vi "DL-SMART-MS-Modify-05-25-5.0.vi"() -> ()   [LabVIEW 2013]
uses:
  <vilib>/Utility/file.llb/Read From Spreadsheet File (DBL).vi
  <vilib>/Utility/file.llb/Write To Spreadsheet File (DBL).vi
  <vilib>/vision/driver/NI_Vision_Acquisition_Software.lvlib
  <resource>/objmgr/imaqdx.rc
panel:
  in  "Shots/Point":i32=100
  in  "chamber in":bool caption="TakeMS"
  in  "chamber out":bool caption="TakeMS"
  out "Mass Spectrum (质谱图)":cluster{i32[], dbl[]}(graph)
  out "Image":T1(plugin-control)
  in  "Laser parameter":T3
  in  "ADC parameter":T4
  in  "ShutDownSystem":bool
  out "TenAccumulate":cluster{"MassX":dbl[], "TenScans":sgl[]}
  in  "ADC reference":refnum<vi>
  in  "SetLaserEnergy":dbl(slide) min=0.0 max=50.0 scale=0.0..20.0
  in  "LaserHV":u8=50 min=1 max=100
  in  "频率/Hz":u8=60
  out "plat zeroed":bool
  out "ADC aquiring":bool
  out "motor moving":bool
  out "busy":bool
  out "Pul.HV-Real":dbl
  in  "ReportResult":bool
  out "Identify Spcetrum":cluster{"all rows":dbl[], "all rows":dbl[]}[](graph)=[{"all rows"=array[50131 elements], "all rows"=array[50131 elements]}, {"all rows"=array[360 elements], "all rows"=[0.0, -15.85746, 0.0, 0.0, -4.11823, 0.0, 0.0, -20.55303, 0.0, 0.0, -3.65583, 0.0, 0.0, -2.69345, 0.0, 0.0, -4.4706, 0.0, 0.0, -6.07537, 0.0, 0.0, -4.25015, 0.0, 0.0, -6.95758, 0.0, 0.0, -2.04252, 0.0, 0.0, -7.70754, 0.0, 0.0, -4.28864, 0.0, 0.0, -4.00869, 0.0, 0.0, -4.47517, 0.0, 0.0, -14.21368, 0.0, 0.0, -6.66072, 0.0, 0.0, -6.50078, 0.0, 0.0, -3.75903, 0.0, 0.0, -17.29715, 0.0, 0.0, -6.92254, 0.0, 0.0, -2.52353, 0.0, 0.0, -3.06405, 0.0, 0.0, -16.54211, 0.0, 0.0, -5.10076, 0.0, 0.0, -8.01669, 0.0, 0.0, -40.71695, 0.0, 0.0, -4.03763, 0.0, 0.0, -3.14159, 0.0, 0.0, -2.79298, 0.0, 0.0, -13.41979, 0.0, 0.0, -7.6464, 0.0, 0.0, -6.18956, 0.0, 0.0, -2.44901, 0.0, 0.0, -5.1704, 0.0, 0.0, -3.62455, 0.0, 0.0, -6.443, 0.0, 0.0, -24.18432, 0.0, 0.0, -37.78631, 0.0, 0.0, -4.28528, 0.0, 0.0, -3.21654, 0.0, 0.0, -3.13522, 0.0, 0.0, -4.8477, 0.0, 0.0, -3.80614, 0.0, 0.0, -8.10386, 0.0, 0.0, -2.86382, 0.0, 0.0, -17.8978, 0.0, 0.0, -4.74503, 0.0, 0.0, -9.4855, 0.0, 0.0, -5.75364, 0.0, 0.0, -80.29859, 0.0, 0.0, -5.18928, 0.0, 0.0, -28.13783, 0.0, 0.0, -6.84449, 0.0, 0.0, -4.07742, 0.0, 0.0, -2.99391, 0.0, 0.0, -4.60838, 0.0, 0.0, -3.257, 0.0, 0.0, -5.79015, 0.0, 0.0, -24.98325, 0.0, 0.0, -4.30828, 0.0, 0.0, -5.54625, 0.0, 0.0, -5.47663, 0.0, 0.0, -100.0001, 0.0, 0.0, -21.11295, 0.0, 0.0, -12.03347, 0.0, 0.0, -6.35092, 0.0, 0.0, -4.71483, 0.0, 0.0, -6.58836, 0.0, 0.0, -3.41548, 0.0, 0.0, -3.10072, 0.0, 0.0, -4.79955, 0.0, 0.0, -4.88109, 0.0, 0.0, -32.02295, 0.0, 0.0, -20.17071, 0.0, 0.0, -9.63953, 0.0, 0.0, -8.63946, 0.0, 0.0, -6.018, 0.0, 0.0, -6.3389, 0.0, 0.0, -14.67808, 0.0, 0.0, -6.22948, 0.0, 0.0, -4.9166, 0.0, 0.0, -44.64096, 0.0, 0.0, -5.6163, 0.0, 0.0, -8.56872, 0.0, 0.0, -11.1186, 0.0, 0.0, -4.42493, 0.0, 0.0, -15.45284, 0.0, 0.0, -2.99091, 0.0, 0.0, -18.05376, 0.0, 0.0, -3.06669, 0.0, 0.0, -35.88844, 0.0, 0.0, -19.12645, 0.0, 0.0, -3.20878, 0.0, 0.0, -2.61247, 0.0, 0.0, -7.79975, 0.0, 0.0, -5.8874, 0.0, 0.0, -5.7487, 0.0, 0.0, -5.43834, 0.0, 0.0, -21.69908, 0.0, 0.0, -64.96584, 0.0, 0.0, -5.77762, 0.0, 0.0, -5.55465, 0.0, 0.0, -4.62119, 0.0, 0.0, -3.61176, 0.0, 0.0, -6.99332, 0.0, 0.0, -4.34549, 0.0, 0.0, -15.09003, 0.0, 0.0, -6.25437, 0.0, 0.0, -21.85243, 0.0, 0.0, -13.24381, 0.0, 0.0, -3.94672, 0.0, 0.0, -3.90192, 0.0, 0.0, -11.14967, 0.0, 0.0, -83.69183, 0.0, 0.0, -11.19559, 0.0, 0.0, -7.83445, 0.0, 0.0, -3.14763, 0.0, 0.0, -6.44728, 0.0, 0.0, -5.69155, 0.0, 0.0, -4.00216, 0.0]}]
  in  "IdentifyMS":bool
  in  "Identification Record (鉴定记录表)":i32(listbox)=6
  in  "Identification Results (单靶鉴定结果)":i32(listbox)=2
  in  "HVEnable":bool
  out "执行进度栏":u8(slide) caption="Vaccum" scale=0.0..1.0
  out "GateClose":bool
  out "LaserOK":bool
  out "HV-OK":bool
  out "Vacuum-OK":bool
  in  "Tab Control":T5(tab)
  in  "helix-Zeta-Step":dbl=100.0
  in  "helix-b":dbl=0.2
  in  "AcquireMS-Methods":u8(ring) items=["SinglePoint", "Multipoints", "MultiTar"]
  in  "MCPHV-Set":dbl=1400.0 min=0.0 max=1600.0
  in  "LensHV-Set":dbl=8000.0 min=0.0 max=10000.0
  in  "Tar.HV-Set":dbl=18010.0 min=0.0 max=20000.0
  in  "Pul.HV-Set":dbl=1400.0 min=0.0 max=2000.0
  in  "PulseDelay":dbl
  in  "ADCFreq":dbl
  in  "CH1_Coupling":u64(ring)=2 items=["Volt DC"=1, "Volt AC"=2, "Ampere DC"=4, "Ampere AC"=8, "Ohm"=16]
  in  "Channel 1_Range":dbl(ring)=4.0 items=["80 V"=80.0, "40 V"=40.0, "20 V"=20.0, "8 V"=8.0, "4 V"=4.0, "2 V"=2.0, "800 mV"=0.8, "400 mV"=0.4, "200 mV"=0.2]
  in  "Anal. Setting File":string="High Mass"
  in  "SettingFileSave":bool caption="TakeMS"
  in  "SettingFileAppl":bool caption="TakeMS"
  in  "SettingDel":bool caption="TakeMS"
  in  "RunADC":bool caption="TakeMS"
  out "ADCstatus":bool
  in  "Vac_Prot.":bool
  in  "Turbo_Fore":bool
  in  "Main_Samp":bool
  in  "Samp_Atmos":bool
  in  "Fore_Samp":bool
  in  "StartPump":bool
  in  "SopPump":bool
  out "TurboSpeed":dbl(knob) scale=0.0..100.0
  out "PumpKW":dbl
  out "PumpAmps":dbl
  out "PumpTemp":u16
  out "PumpVolts":dbl
  in  "laser OFF":bool
  in  "laser ON":bool
  out "cluster":T6
  out "A1-position-Y":dbl=45.0 caption="Y" min=0.0 max=55.0
  out "A1-position-X":dbl=53.4 caption="X" min=0.0 max=55.0
  in  "GO":bool
  in  "Y":dbl min=0.0 max=55.0
  in  "X":dbl min=0.0 max=55.0
  in  "A1-Position":bool caption="X-"
  in  "Plat_To_Zero":bool caption="TakeMS"
  in  "Plat_Cal":bool caption="TakeMS"
  out "Ty":dbl
  out "Tx":dbl
  out "Y当前":dbl
  out "X当前":dbl
  out "移动":bool
  out "Y满":bool
  out "Y标":bool
  out "X满":bool
  out "Y0":bool
  out "X0":bool
  out "靶位In/Out":bool
  out "仓门":bool
  out "Y过热":bool
  out "X过热":bool
  out "通讯":bool
  in  "Operation Record":i32(listbox)
  in  "OptionRecordLoad 2":bool caption="TakeMS"
  in  "OptionRecordClear":bool caption="TakeMS"
  out "Tar.HV-Real":dbl
  out "LensHV-Real":dbl
  out "MCPHV-Real":dbl
  out "Lvaccum":dbl=0.83 format="%#_2e"
  out "Hvaccum":dbl=3.4e-05 format="%#_2e"
  in  "H12":bool
  in  "G12":bool
  in  "F12":bool
  in  "E12":bool
  in  "D12":bool
  in  "C12":bool
  in  "B12":bool
  in  "A12":bool
  in  "H11":bool
  in  "G11":bool
  in  "F11":bool
  in  "E11":bool
  in  "D11":bool
  in  "C11":bool
  in  "B11":bool
  in  "A11":bool
  in  "H10":bool
  in  "G10":bool
  in  "F10":bool
  in  "E10":bool
  in  "D10":bool
  in  "C10":bool
  in  "B10":bool
  in  "A10":bool
  in  "H9":bool
  in  "G9":bool
  in  "F9":bool
  in  "E9":bool
  in  "D9":bool
  in  "C9":bool
  in  "B9":bool
  in  "A9":bool
  in  "H8":bool
  in  "G8":bool
  in  "F8":bool
  in  "E8":bool
  in  "D8":bool
  in  "C8":bool
  in  "B8":bool
  in  "A8":bool
  in  "H7":bool
  in  "G7":bool
  in  "F7":bool
  in  "E7":bool
  in  "D7":bool
  in  "C7":bool
  in  "B7":bool
  in  "A7":bool
  in  "H6":bool
  in  "G6":bool
  in  "F6":bool
  in  "E6":bool
  in  "D6":bool
  in  "C6":bool
  in  "B6":bool
  in  "A6":bool
  in  "H5":bool
  in  "G5":bool
  in  "F5":bool
  in  "E5":bool
  in  "D5":bool
  in  "C5":bool
  in  "B5":bool
  in  "A5":bool
  in  "H4":bool
  in  "G4":bool
  in  "F4":bool
  in  "E4":bool
  in  "D4":bool
  in  "C4":bool
  in  "B4":bool
  in  "A4":bool
  in  "H3":bool
  in  "G3":bool
  in  "F3":bool
  in  "E3":bool
  in  "D3":bool
  in  "C3":bool
  in  "B3":bool
  in  "A3":bool
  in  "H2":bool
  in  "G2":bool
  in  "F2":bool
  in  "E2":bool
  in  "D2":bool
  in  "C2":bool
  in  "B2":bool
  in  "A2":bool
  in  "H1":bool
  in  "G1":bool
  in  "F1":bool
  in  "E1":bool
  in  "D1":bool
  in  "C1":bool
  in  "B1":bool
  in  "A1":bool
  in  "Clear":bool caption="TakeMS"
  in  "Add":bool caption="TakeMS"
  in  "TakeMS-Stop":bool caption="TakeMS"
  in  "TakeMS-Run":bool caption="TakeMS"
  # "Camera (摄像头)"
  # "Laser (激光)"
  # "Acq.(采谱)"
  # "Vacuum(真空)"
  # "Pa"
  # "High"
  # "1"
  # "2"
  # "3"
  # "4"
  # "5"
  # "6"
  # "7"
  # "8"
  # "9"
  # "10"
  # "11"
  # "12"
  # "A"
  # "Low"
  # "Pa"
  # "B"
  # "H.V.(高压)"
  # "C"
  # "D"
  # "Ident. (鉴定图)"
  # "MCP"
  # "V"
  # "E"
  # "Tar."
  # "V"
  # "F"
  # "Pul."
  # "V"
  # "G"
  # "Lens"
  # "V"
  # "H"
  # "Vauum (真空)"
  # "H.V. (高压)"
  # "Laser (激光)"
  # "Gate (仓门)"
  # "mm"
  # "Radian"
  # "H.V. (高压参数)"
  # "ADC(采集卡设置)"
  # "ADCFreq(采样)"
  # "MCP (探测器)"
  # "V"
  # "Hz"
  # "Tar. (靶)"
  # "V"
  # "Setting File(设置文件)"
  # "Coupling"
  # "Pulse (脉冲)"
  # "V"
  # "IntRange"
  # "V"
  # "Lens (透镜)"
  # "Delay (延时)"
  # "ns"
  # "Sole. Valves"
  # "Turbo Pump"
  # "自锁保护"
  # "机械/分子"
  # "主仓/样仓"
  # "样仓/大气"
  # "机械/样仓"
  # "激光器状态"
  # "mm"
  # "mm"
  # "mm"
  # "mm"
  # "mm"
  # "mm"
  # "度"
  # "度"
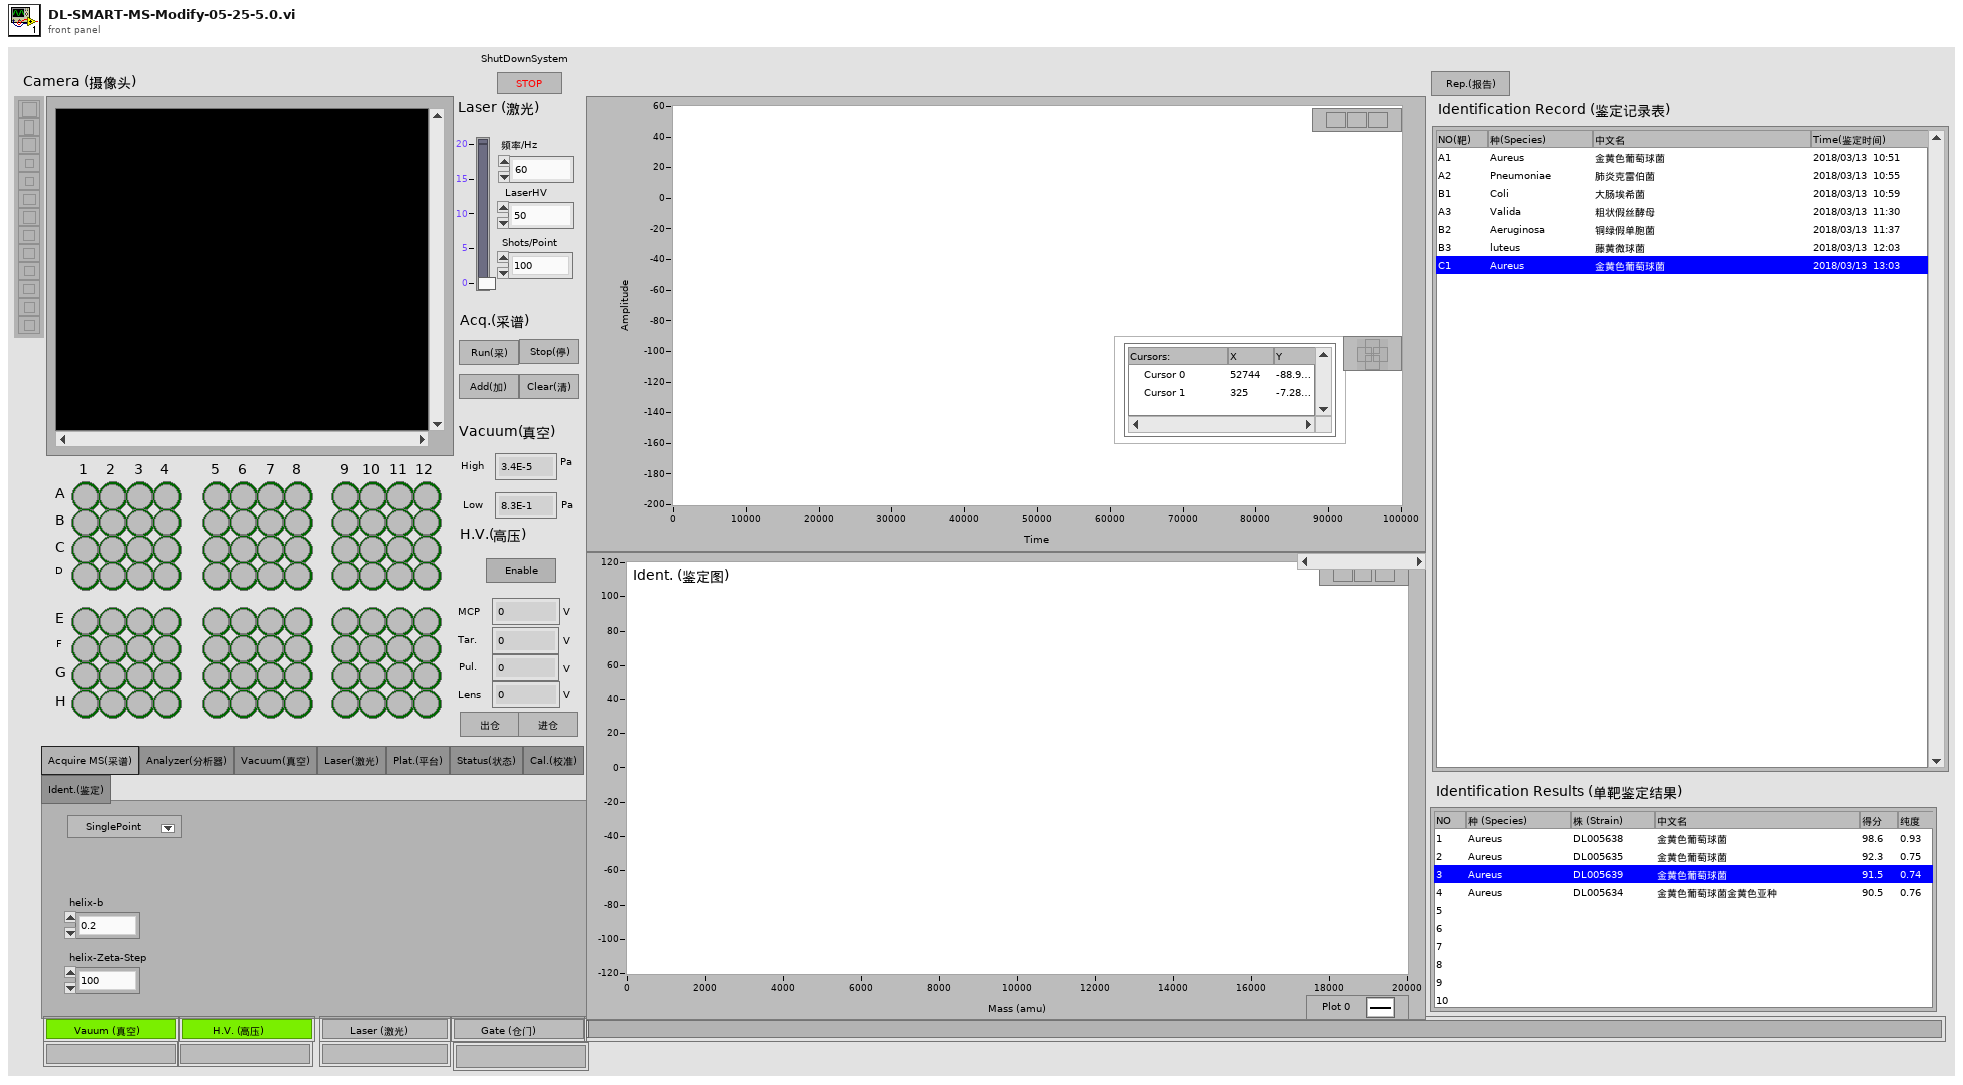
[diagram p1: front panel]
types:
  T1 = typedef "IMAQ Image.ctl" = refnum<image>
  T2 = typedef "Semaphore RefNum" = refnum<k1>
  T3 = cluster{"VISA resource name":refnum<visa-resource-name>, "standby":bool, "semaphore in":T2, "SetLaserEnergy":dbl}
  T4 = cluster{"TpDeviceHandle_t":u32, "Record Length/Samples":u64, "ShotsPerPoint":u16}
  T5 = enum32{"Acquire MS(采谱)", "Analyzer(分析器)", "Vacuum(真空)", "Laser(激光)", "Plat.(平台)", "Status(状态)", "Cal.(校准)", "Ident.(鉴定)"}
  T6 = cluster{"链接":bool, "待机":bool, "发射":bool, "[3]":bool, "内存":bool, "测能":bool, "温警":bool, "静态":bool, "操作":bool}
  T7 = cluster{"laser semaphore":T2, "pump semaphore":T2}
  T8 = enum8{"Enabled", "Disabled", "Disabled and Grayed Out"}
  T9 = cluster{"monitor":refnum<user-event>, "motor status":refnum<user-event>, "motor":refnum<user-event>, "notifier out":refnum<notifier>, "queue out":refnum<queue>, "AI":T2, "DI":T2, "CX":T2, "CY":T2}
  T10 = cluster{"AI Task":refnum<k21>, "AO Task":refnum<k21>, "DO Task":refnum<k21>, "DI Task":refnum<k21>, "PWM x":refnum<k21>, "PWM y":refnum<k21>, "counter x":refnum<k21>, "counter y":refnum<k21>}
  T11 = cluster{"tasks":cluster{"AI Task":refnum<k21>, "AO Task":refnum<k21>, "DO Task":refnum<k21>, "DI Task":refnum<k21>, "PWM x":refnum<k21>, "PWM y":refnum<k21>, "counter x":refnum<k21>, "counter y":refnum<k21>}, "interface":cluster{"monitor":refnum<user-event>, "motor status":refnum<user-event>, "motor":refnum<user-event>, "notifier out":refnum<notifier>, "queue out":refnum<queue>, "AI":T2, "DI":T2, "CX":T2, "CY":T2}, "error out":errorcluster}
  T12 = cluster{"ConfiguredPumpCom":refnum<visa-resource-name>, "ConfiguredLaserCom":refnum<visa-resource-name>}
  T13 = typedef "LVPoint32TypeDef.ctl" = cluster{"Horizontal":i32, "Vertical":i32}
  T14 = cluster{"Type":u32, "Version":u32, "Flags":u32, "SerialNumberHigh":u32, "SerialNumberLow":u32, "BusType":u32, "InterfaceName":string, "VendorName":string, "ModelName":string, "CameraFileName":string, "CameraAttributeURL":string}[]
  T15 = cluster{"Type":u32, "Version":u32, "Flags":u32, "SerialNumberHigh":u32, "SerialNumberLow":u32, "BusType":u32, "InterfaceName":string, "VendorName":string, "ModelName":string, "CameraFileName":string, "CameraAttributeURL":string}
  T16 = typedef "IMAQdx.ctl" = refnum<k21>
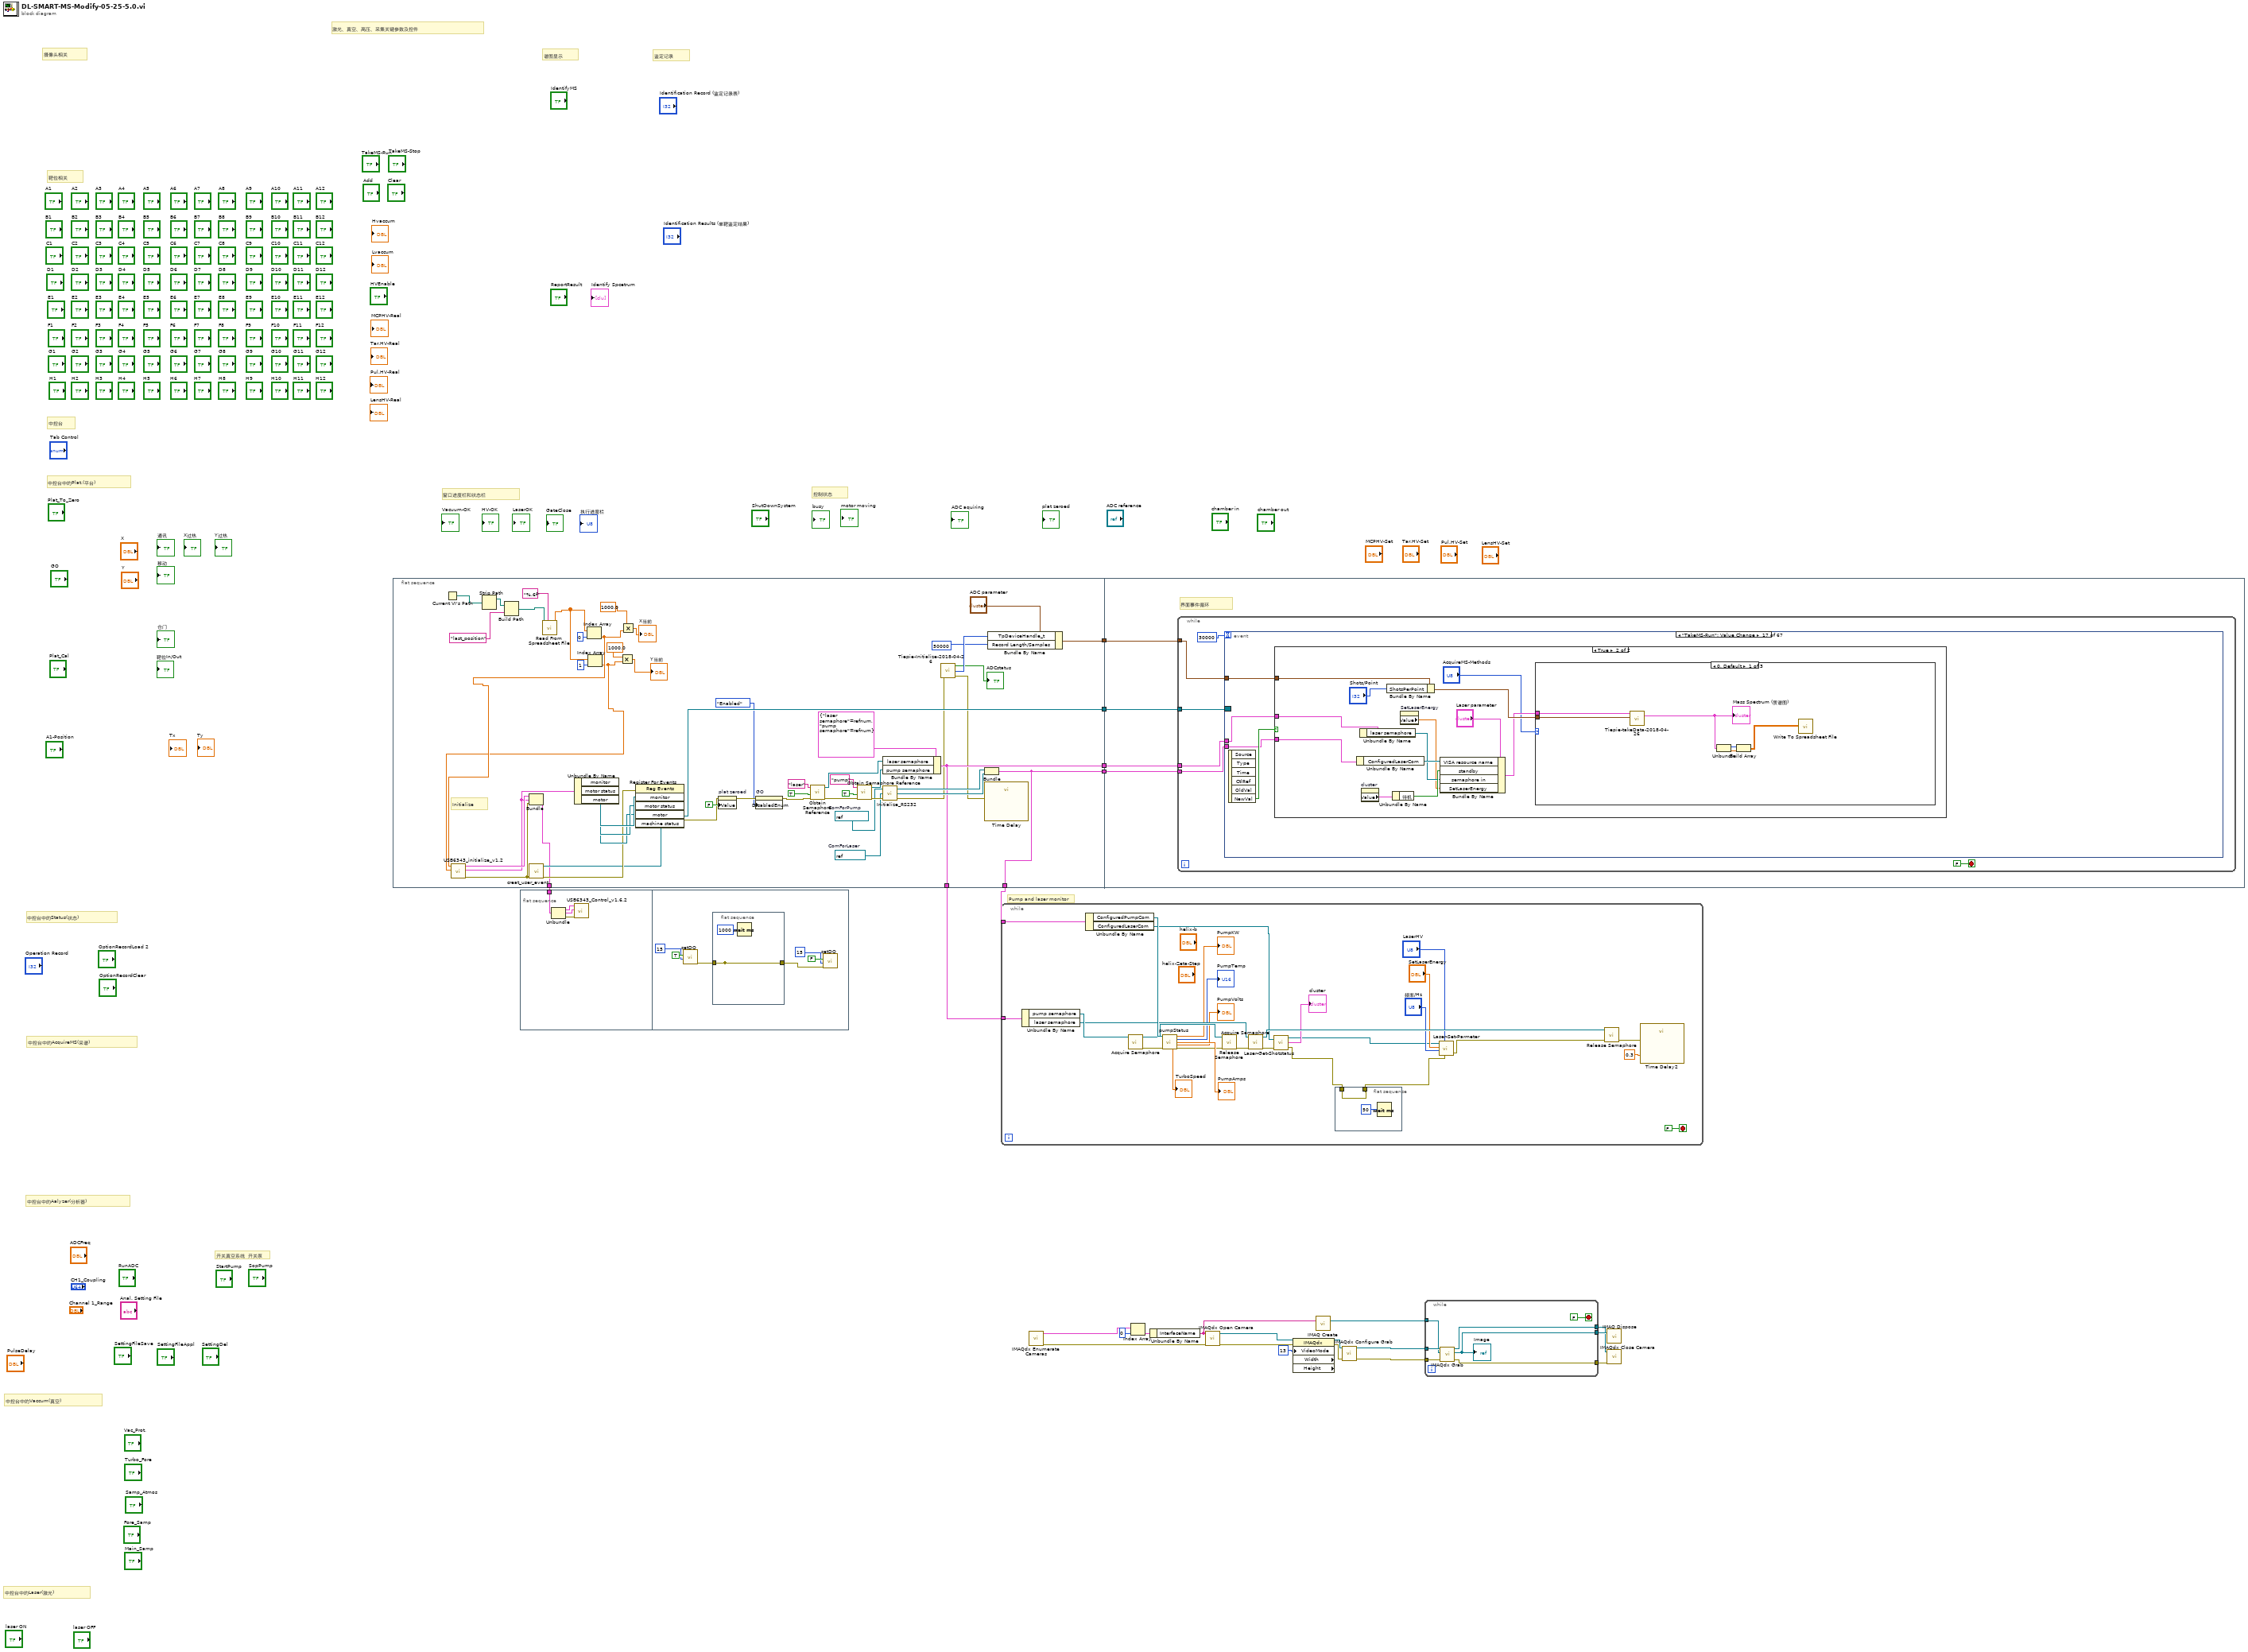
[diagram p0: block diagram]
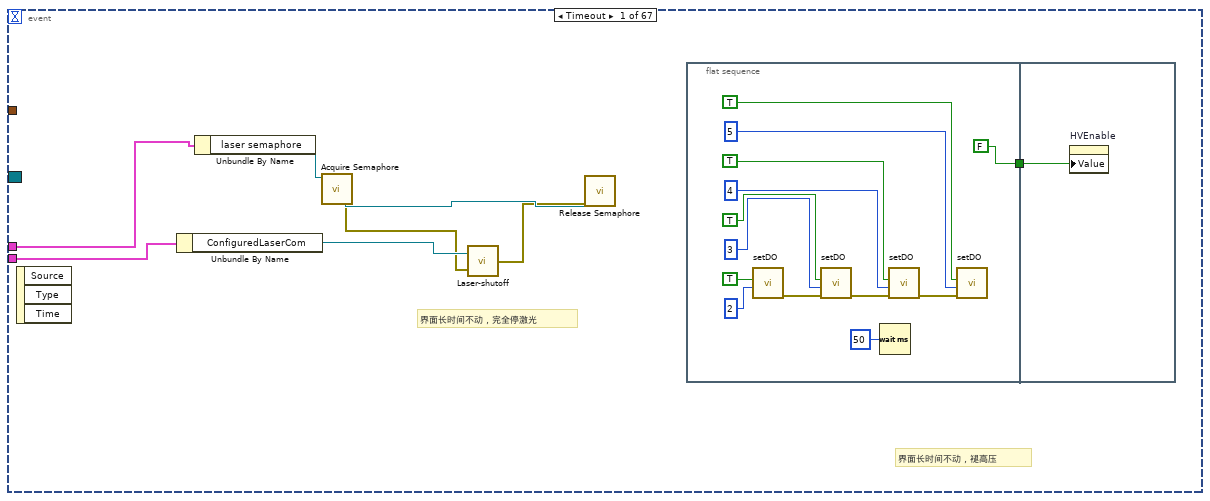
[diagram p2: hidden frame]
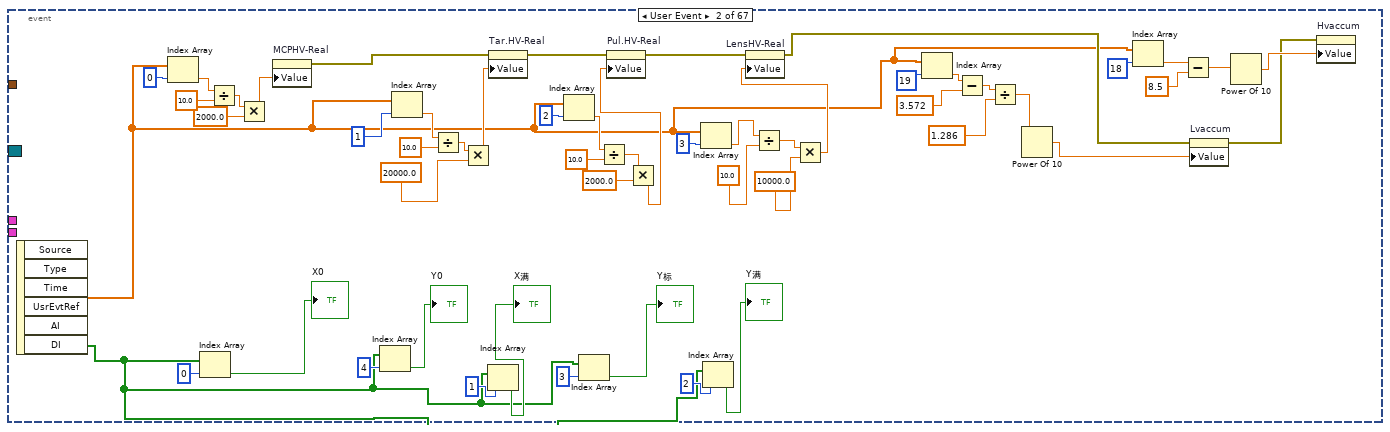
[diagram p3: hidden frame]
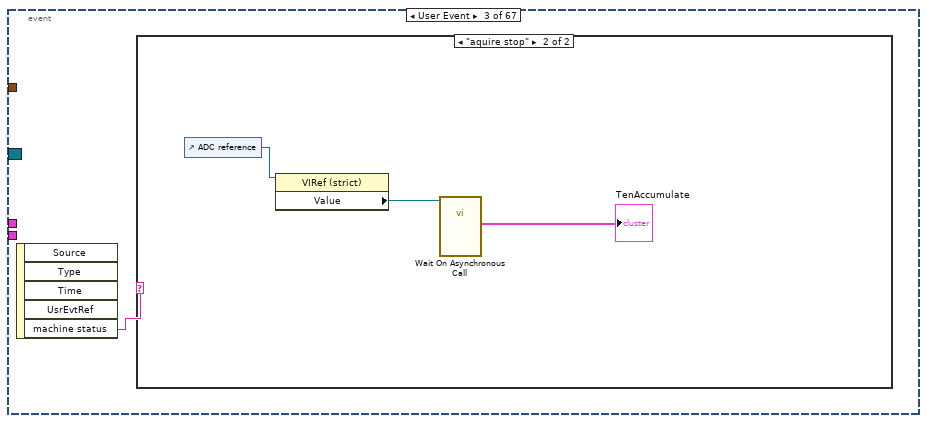
[diagram p4: hidden frame]
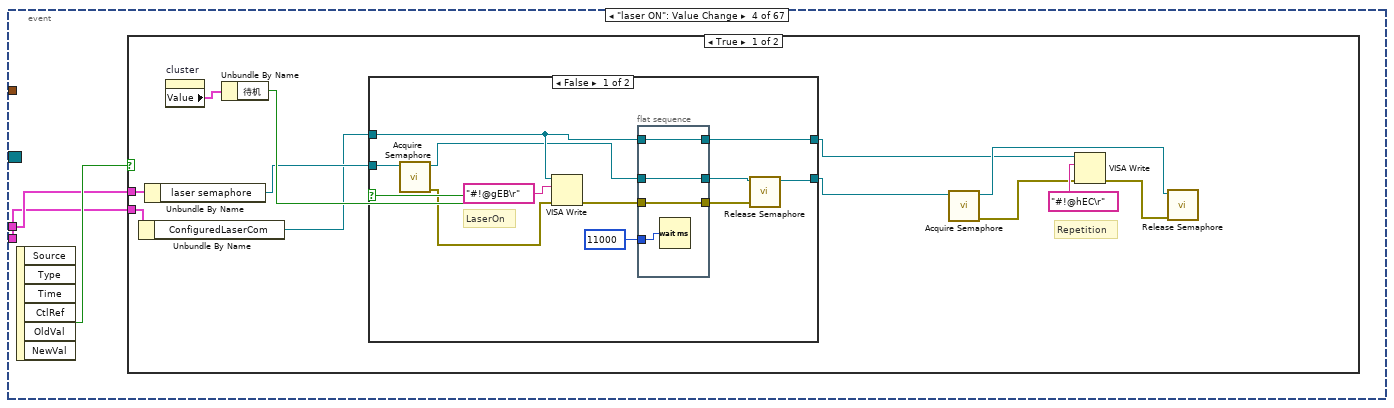
[diagram p6: hidden frame]
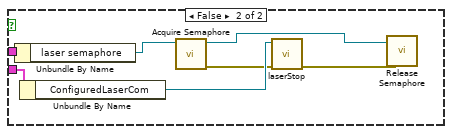
[diagram p8: hidden frame]
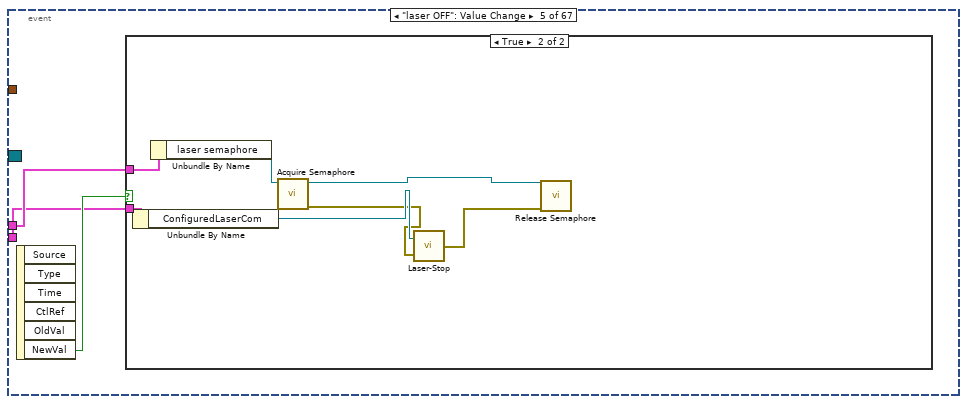
[diagram p9: hidden frame]
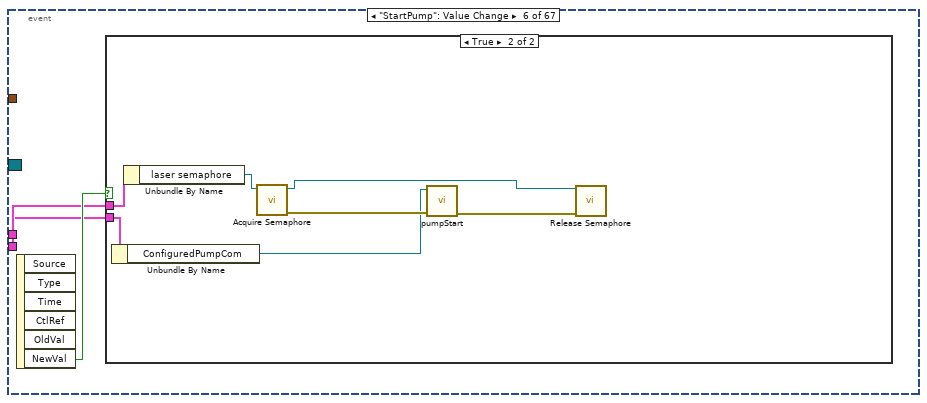
[diagram p11: hidden frame]
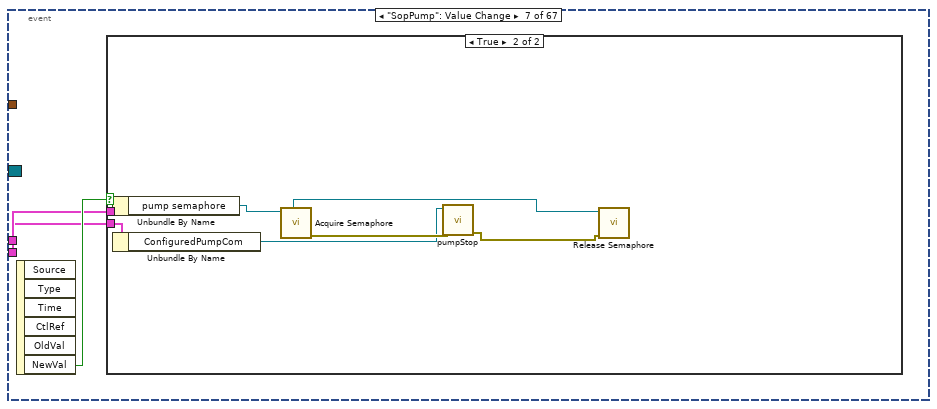
[diagram p13: hidden frame]
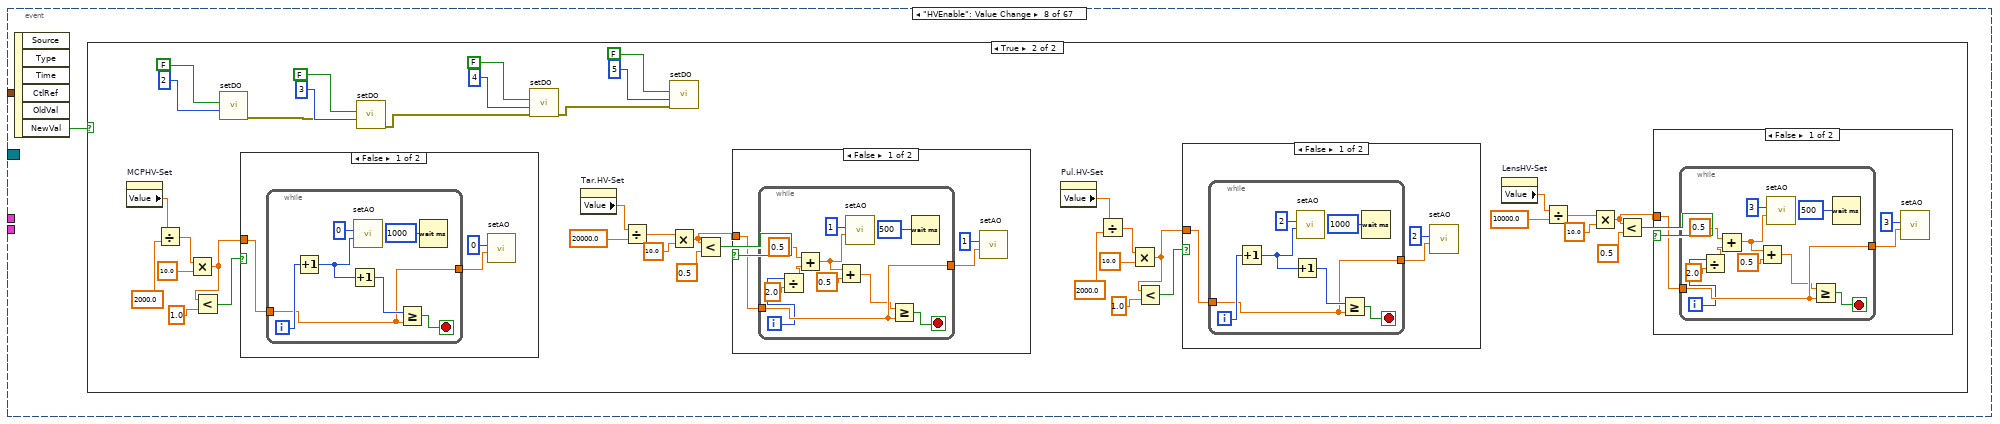
[diagram p15: hidden frame]
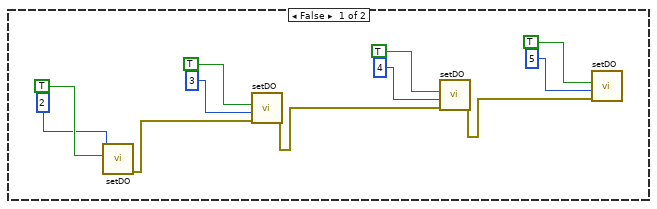
[diagram p16: hidden frame]
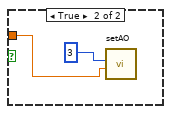
[diagram p17: hidden frame]
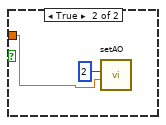
[diagram p18: hidden frame]
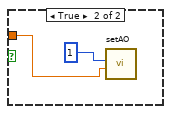
[diagram p19: hidden frame]
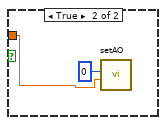
[diagram p20: hidden frame]
diagram:
  # "Pump and laser monitor"
  # "开关真空系统  开关泵"
  # "控制状态"
  # "鉴定记录"
  # "谱图显示"
  # "激光、真空、高压、采集关键参数及控件"
  # "窗口进度栏和状态栏"
  # "中控台中的Laser(激光)"
  # "中控台中的Vaccum(真空)"
  # "中控台中的Aalyzer(分析器)"
  # "中控台中的AcquireMS(采谱)"
  # "中控台中的Status(状态)"
  # "中控台中的Plat.(平台)"
  # "中控台"
  # "靶位相关"
  # "摄像头相关"
  n1 = flat-sequence {
    tunnel: [w71] -> w23
    tunnel: [w48] -> w22
    tunnel: [w48] -> w20
    tunnel: [w47] -> w21
    tunnel: [w47] -> w19
    tunnel: [w51] -> w18
    tunnel: [w39] -> w17
    tunnel: w23 -> [w78]
    tunnel: w22 -> [w77]
    tunnel: w21 -> [w76]
    tunnel: w17 -> [w75]
    frame #0 {
      w45 = refnum<visa-resource-name> "COM9"  # ComForLaser
      w46 = refnum<visa-resource-name> "COM10"  # ComForPump
      # "Initialize"
      n2 = Current VI's Path() -> (path=w37:path)
      n3 = Strip Path(path=w37) -> (stripped path=w36:path)  [unwired: 1 out]
      n4 = Build Path(base path=w36, name or relative path="last_position") -> (appended path=w34:path)
      n5 = call-poly <vilib>:"Read From Spreadsheet File.vi"("format (%.3f)"="%.6f", "file path (dialog if empty)"=w34) -> ("first row"=w32:dbl[])  [unwired: 5 in, 4 out]
      n6 = Index Array(array=w32, index=0) -> (element=w29:dbl)
      n7 = Index Array(array=w32, index=1) -> (element=w26:dbl)
      n8 = call "USB6343_initialize_v1.2.vi"("Y initial position"=w26, "X initial position"=w29) -> ("error out"=w52:errorcluster, "interface"=w53:T9, "tasks"=w54:T10)  [unwired: 7 in]
      n9 = Bundle("tasks"=w54, "interface"=w53, "error out"=w52) -> (w51:T11)  [unwired: 1 in]
      n10 = call "creat_user_event.vi"("error in (no error)"=w52) -> ("error out"=w65:errorcluster, "machine status"=w62:refnum<user-event>)  [unwired: 9 in]
      n11 = Unbundle By Name(w53) -> ("monitor"=w74:refnum<user-event>, "motor status"=w73:refnum<user-event>, "motor"=w72:refnum<user-event>)
      n12 = Multiply(x=1000.0, y=w26) -> (x*y=→"Y当前":dbl)
      n13 = Multiply(x=1000.0, y=w29) -> (x*y=→"X当前":dbl)
      n14 = register-events(error in=w65, w74, w73, w72, w62) -> (reference out=w71:refnum<event-registration>, error out=w64:errorcluster)  [unwired: 1 in]
      n15 = property on="plat zeroed" class="Bool (strict)"(error in=w64, "Value"=FALSE ("plat zeroed")) -> (error out=w69:errorcluster)  [unwired: 1 in, 1 out]
      n16 = property on="GO" class="Bool (strict)"(error in=w69, "DisabledEnum"=T8."Enabled" ("Disabled")) -> (error out=w63:errorcluster)  [unwired: 1 in, 1 out]
      n17 = call <vilib>:"Obtain Semaphore Reference.vi"("error in (no error)"=w63, "create if not found (T)"=TRUE, "name (unnamed)"="laser") -> ("error out"=w58:errorcluster, "semaphore"=w55:T2)  [unwired: 2 in, 1 out]
      n18 = call <vilib>:"Obtain Semaphore Reference.vi"("error in (no error)"=w58, "create if not found (T)"=TRUE, "name (unnamed)"="pump") -> ("error out"=w57:errorcluster, "semaphore"=w49:T2)  [unwired: 2 in, 1 out]
      n19 = Bundle By Name(cluster=T7 {"laser semaphore"=refnum, "pump semaphore"=refnum}, "laser semaphore"=w55, "pump semaphore"=w49) -> (w48:T7)
      n20 = call "Initialize_RS232.vi"("error in (no error)"=w57, "ComForLaser"=w45, "ComForPump"=w46) -> ("error out"=w44:errorcluster, "ConfiguredLaserCom"=w60:refnum<visa-resource-name>, "ConfiguredPumpCom"=w61:refnum<visa-resource-name>)
      n21 = call "Tiepie-Initialize-2018-04-26.vi"("error in (no error)"=w44) -> ("error out"=w43:errorcluster, "TpDeviceHandle_t"=w41:u32, "Card-OK"=→"ADCstatus":bool)  [unwired: 3 in]
      n22 = Bundle("ConfiguredPumpCom"=w61, "ConfiguredLaserCom"=w60) -> (w47:T12)  [unwired: 1 in]
      n23 = call "Time Delay"("error in (no error)"=w43) -> ()  [unwired: 10 in, 1 out]
      n24 = Bundle By Name(cluster="ADC parameter", "TpDeviceHandle_t"=w41, "Record Length/Samples"=u64 50000) -> (w39:T4)
    }
    frame #1 {
      # "界面事件循环"
      n25 = while {
        tunnel: w78 -> [w84]
        tunnel: w76 -> [w83]
        tunnel: w77 -> [w82]
        tunnel: w75 -> [w80]
        stop <- FALSE stop-if-true
        n26 = event shown="[16] \"TakeMS-Run\": Value Change" {
          selector: w84 -> [_ _ _ _ _ _ _ _ _ _ _ _ _ _ _ _ _ _ _ _ _ _ _ _ _ _ _ _ _ _ _ _ _ _ _ _ _ _ _ _ _ _ _ _ _ _ _ _ _ _ _ _ _ _ _ _ _ _ _ _ _ _ _ _ _ _ _]
          dyn-events: _ -> [_ _ _ _ _ _ _ _ _ _ _ _ _ _ _ _ _ _ _ _ _ _ _ _ _ _ _ _ _ _ _ _ _ _ _ _ _ _ _ _ _ _ _ _ _ _ _ _ _ _ _ _ _ _ _ _ _ _ _ _ _ _ _ _ _ _ _]
          timeout: 30000 -> [_ _ _ _ _ _ _ _ _ _ _ _ _ _ _ _ _ _ _ _ _ _ _ _ _ _ _ _ _ _ _ _ _ _ _ _ _ _ _ _ _ _ _ _ _ _ _ _ _ _ _ _ _ _ _ _ _ _ _ _ _ _ _ _ _ _ _]
          tunnel: w83 -> [w86 _ _ w164 w203 w213 w223 _ _ _ _ _ _ _ _ _ w421 _ _ _ _ _ _ _ _ _ _ _ _ _ _ _ _ _ _ _ _ _ _ _ _ _ _ _ _ _ _ _ _ _ _ _ _ _ _ _ _ _ _ _ _ _ _ _ _ _ w1243]
          tunnel: w82 -> [w87 _ _ w165 w204 w214 w224 _ _ _ _ _ _ _ _ _ w422 _ _ _ _ _ _ _ _ _ _ _ _ _ _ _ _ _ _ _ _ _ _ _ _ _ _ _ _ _ _ _ _ _ _ _ _ _ _ _ _ _ _ _ _ _ _ _ _ _ _]
          tunnel: w80 -> [_ _ _ _ _ _ _ _ _ _ _ _ _ _ _ _ w423 _ _ _ _ _ _ _ _ _ _ _ _ _ _ _ _ _ _ _ _ _ _ _ _ _ _ _ _ _ _ _ _ _ _ _ _ _ _ _ _ _ _ _ _ _ _ _ _ _ _]
          event Timeout {
            # "界面长时间不动，褪高压"
            # "界面长时间不动，完全停激光"
            n27 = event-data() -> ()  [unwired: 1 in, 3 out]
            n28 = Unbundle By Name(w86) -> ("ConfiguredLaserCom"=w90:refnum<visa-resource-name>)
            n29 = Unbundle By Name(w87) -> ("laser semaphore"=w92:T2)
            n30 = call <vilib>:"Acquire Semaphore.vi"("semaphore"=w92) -> ("error out"=w89:errorcluster, "semaphore out"=w91:T2)  [unwired: 4 in, 1 out]
            n31 = call "Laser-shutoff.vi"("error in (no error)"=w89, "VISA resource name"=w90) -> ("error out"=w88:errorcluster)
            n32 = call <vilib>:"Release Semaphore.vi"("error in (no error)"=w88, "semaphore"=w91) -> ()  [unwired: 4 in, 2 out]
            n33 = flat-sequence {
              tunnel: [FALSE ("HVEnable")] -> w85
              tunnel: w85 -> [w106]
              frame #0 {
                n34 = call "setDO.vi"("channel"=2, "on/off"=TRUE) -> ("错误输出"=w103:errorcluster)  [unwired: 9 in]
                n35 = call "setDO.vi"("错误输入（无错误）"=w103, "channel"=3, "on/off"=TRUE) -> ("错误输出"=w104:errorcluster)  [unwired: 8 in]
                n36 = Wait (ms)(milliseconds to wait=u32 50) -> ()  [unwired: 1 out]
                n37 = call "setDO.vi"("错误输入（无错误）"=w104, "channel"=4, "on/off"=TRUE) -> ("错误输出"=w105:errorcluster)  [unwired: 8 in]
                n38 = call "setDO.vi"("错误输入（无错误）"=w105, "channel"=5, "on/off"=TRUE) -> ()  [unwired: 8 in, 1 out]
              }
              frame #1 {
                n39 = property on="HVEnable" class="Bool (strict)"("Value"=w106) -> ()  [unwired: 2 in, 2 out]
              }
            }
          }
          event User Event {
            n40 = event-data() -> ("AI"=w118:dbl[], "DI"=w143:bool[])  [unwired: 1 in, 4 out]
            n41 = Index Array(array=w118, index=0) -> (element=w141:dbl)
            n42 = Index Array(array=w143, index=0) -> (element=→"X0":bool)
            n43 = Divide(x=w141, y=10.0) -> (x/y=w139:dbl)
            n44 = Multiply(x=w139, y=2000.0) -> (x*y=w137:dbl)
            n45 = property on="MCPHV-Real" class="DigNum (strict)"("Value"=w137) -> (error out=w159:errorcluster)  [unwired: 2 in, 1 out]
            n46 = Index Array(array=w143, index=4) -> (element=→"Y0":bool)
            n47 = Index Array(array=w118, index=1) -> (element=w136:dbl)
            n48 = Divide(x=w136, y=10.0) -> (x/y=w134:dbl)
            n49 = Multiply(x=w134, y=20000.0) -> (x*y=w132:dbl)
            n50 = Index Array(array=w143, index=1) -> (element=→"X满":bool)
            n51 = property on="Tar.HV-Real" class="DigNum (strict)"(error in=w159, "Value"=w132) -> (error out=w158:errorcluster)  [unwired: 1 in, 1 out]
            n52 = Index Array(array=w118, index=2) -> (element=w131:dbl)
            n53 = Index Array(array=w143, index=3) -> (element=→"Y标":bool)
            n54 = Divide(x=w131, y=10.0) -> (x/y=w129:dbl)
            n55 = Multiply(x=w129, y=2000.0) -> (x*y=w127:dbl)
            n56 = property on="Pul.HV-Real" class="DigNum (strict)"(error in=w158, "Value"=w127) -> (error out=w157:errorcluster)  [unwired: 1 in, 1 out]
            n57 = Index Array(array=w118, index=3) -> (element=w126:dbl)
            n58 = Index Array(array=w143, index=2) -> (element=→"Y满":bool)
            n59 = Divide(x=w126, y=10.0) -> (x/y=w124:dbl)
            n60 = Multiply(x=w124, y=10000.0) -> (x*y=w122:dbl)
            n61 = property on="LensHV-Real" class="DigNum (strict)"(error in=w157, "Value"=w122) -> (error out=w120:errorcluster)  [unwired: 1 in, 1 out]
            n62 = Index Array(array=w118, index=19) -> (element=w117:dbl)
            n63 = Subtract(x=w117, y=3.572) -> (x-y=w115:dbl)
            n64 = Divide(x=w115, y=1.286) -> (x/y=w113:dbl)
            n65 = Power Of 10(x=w113) -> (10^x=w112:dbl)
            n66 = Index Array(array=w118, index=18) -> (element=w111:dbl)
            n67 = Subtract(x=w111, y=8.5) -> (x-y=w109:dbl)
            n68 = property on="Lvaccum" class="DigNum (strict)"(error in=w120, "Value"=w112) -> (error out=w107:errorcluster)  [unwired: 1 in, 1 out]
            n69 = Power Of 10(x=w109) -> (10^x=w108:dbl)
            n70 = property on="Hvaccum" class="DigNum (strict)"(error in=w107, "Value"=w108) -> ()  [unwired: 1 in, 2 out]
          }
          event User Event {
            n71 = event-data() -> ("machine status"=w160:string)  [unwired: 1 in, 4 out]
            n72 = case shown="\"aquire stop\"" w160 {
              frame "aquire start", Default {
              }
              frame "aquire stop" {
                n73 = control-ref of="ADC reference"() -> (w163:refnum<vi>)
                n74 = property class="VIRef (strict)"(reference=w163) -> ("Value"=w162:refnum<vi>)  [unwired: 1 in, 2 out]
                n75 = call-by-ref "Wait On Asynchronous Call"(reference=w162) -> ("TenAccumulate"=→"TenAccumulate":cluster{"MassX":dbl[], "TenScans":sgl[]})  [unwired: 12 in, 2 out]
              }
            }
          }
          event "laser ON": Value Change {
            n76 = event-data() -> ("NewVal"=w166:bool)  [unwired: 1 in, 5 out]
            n77 = case shown="True" w166 {
              tunnel: w165 -> [w178 w202]
              tunnel: w164 -> [w177 w200]
              frame True {
                # "Repetition"
                n78 = Unbundle By Name(w177) -> ("ConfiguredLaserCom"=w173:refnum<visa-resource-name>)
                n79 = Unbundle By Name(w178) -> ("laser semaphore"=w174:T2)
                n80 = property on="cluster" class="Clust (strict)"() -> ("Value"=w176:T6)  [unwired: 2 in, 2 out]
                n81 = Unbundle By Name(w176) -> ("待机"=w175:bool)
                n82 = case shown="False" w175 {
                  tunnel: w174 -> [w188 w194]
                  tunnel: w173 -> [w185 w195]
                  tunnel: [w181 w194] -> w171
                  tunnel: [w184 w195] -> w167
                  frame False {
                    # "LaserOn"
                    n83 = call <vilib>:"Acquire Semaphore.vi"("semaphore"=w188) -> ("error out"=w187:errorcluster, "semaphore out"=w183:T2)  [unwired: 4 in, 1 out]
                    n84 = VISA Write(VISA resource name=w185, write buffer="#!@gEB\r", error in (no error)=w187) -> (error out=w180:errorcluster)  [unwired: 2 out]
                    n85 = flat-sequence {
                      tunnel: 11000 -> [w193]
                      tunnel: w183 -> [w192]
                      tunnel: [w192] -> w182
                      tunnel: w180 -> [w191]
                      tunnel: [w191] -> w179
                      tunnel: w185 -> [w190]
                      tunnel: [w190] -> w184
                      frame #0 {
                        n86 = Wait (ms)(milliseconds to wait=w193) -> ()  [unwired: 1 out]
                      }
                    }
                    n87 = call <vilib>:"Release Semaphore.vi"("error in (no error)"=w179, "semaphore"=w182) -> ("semaphore out"=w181:T2)  [unwired: 4 in, 1 out]
                  }
                  frame True {
                  }
                }
                n88 = call <vilib>:"Acquire Semaphore.vi"("semaphore"=w171) -> ("error out"=w169:errorcluster, "semaphore out"=w170:T2)  [unwired: 4 in, 1 out]
                n89 = VISA Write(VISA resource name=w167, write buffer="#!@hEC\r", error in (no error)=w169) -> (error out=w168:errorcluster)  [unwired: 2 out]
                n90 = call <vilib>:"Release Semaphore.vi"("error in (no error)"=w168, "semaphore"=w170) -> ()  [unwired: 4 in, 2 out]
              }
              frame False {
                n91 = Unbundle By Name(w202) -> ("laser semaphore"=w201:T2)
                n92 = Unbundle By Name(w200) -> ("ConfiguredLaserCom"=w199:refnum<visa-resource-name>)
                n93 = call <vilib>:"Acquire Semaphore.vi"("semaphore"=w201) -> ("error out"=w198:errorcluster, "semaphore out"=w196:T2)  [unwired: 4 in, 1 out]
                n94 = call "laserStop.vi"("error in (no error)"=w198, "VISA resource name"=w199) -> ("error out"=w197:errorcluster)  [unwired: 9 in]
                n95 = call <vilib>:"Release Semaphore.vi"("error in (no error)"=w197, "semaphore"=w196) -> ()  [unwired: 4 in, 2 out]
              }
            }
          }
          event "laser OFF": Value Change {
            n96 = event-data() -> ("NewVal"=w205:bool)  [unwired: 1 in, 5 out]
            n97 = case shown="True" w205 {
              tunnel: w204 -> [_ w212]
              tunnel: w203 -> [_ w210]
              frame False {
              }
              frame True {
                n98 = Unbundle By Name(w210) -> ("ConfiguredLaserCom"=w208:refnum<visa-resource-name>)
                n99 = Unbundle By Name(w212) -> ("laser semaphore"=w211:T2)
                n100 = call <vilib>:"Acquire Semaphore.vi"("semaphore"=w211) -> ("error out"=w207:errorcluster, "semaphore out"=w209:T2)  [unwired: 4 in, 1 out]
                n101 = call "Laser-Stop.vi"("error in (no error)"=w207, "VISA resource name"=w208) -> ("error out"=w206:errorcluster)
                n102 = call <vilib>:"Release Semaphore.vi"("error in (no error)"=w206, "semaphore"=w209) -> ()  [unwired: 4 in, 2 out]
              }
            }
          }
          event "StartPump": Value Change {
            n103 = event-data() -> ("NewVal"=w215:bool)  [unwired: 1 in, 5 out]
            n104 = case shown="True" w215 {
              tunnel: w214 -> [_ w220]
              tunnel: w213 -> [_ w219]
              frame False {
              }
              frame True {
                n105 = Unbundle By Name(w219) -> ("ConfiguredPumpCom"=w218:refnum<visa-resource-name>)
                n106 = Unbundle By Name(w220) -> ("laser semaphore"=w217:T2)
                n107 = call <vilib>:"Acquire Semaphore.vi"("semaphore"=w217) -> ("error out"=w222:errorcluster, "semaphore out"=w216:T2)  [unwired: 4 in, 1 out]
                n108 = call "pumpStart.vi"("error in (no error)"=w222, "VISA resource name"=w218) -> ("error out"=w221:errorcluster)  [unwired: 9 in]
                n109 = call <vilib>:"Release Semaphore.vi"("error in (no error)"=w221, "semaphore"=w216) -> ()  [unwired: 4 in, 2 out]
              }
            }
          }
          event "SopPump": Value Change {
            n110 = event-data() -> ("NewVal"=w225:bool)  [unwired: 1 in, 5 out]
            n111 = case shown="True" w225 {
              tunnel: w224 -> [_ w229]
              tunnel: w223 -> [_ w227]
              frame False {
              }
              frame True {
                n112 = Unbundle By Name(w229) -> ("pump semaphore"=w228:T2)
                n113 = Unbundle By Name(w227) -> ("ConfiguredPumpCom"=w226:refnum<visa-resource-name>)
                n114 = call <vilib>:"Acquire Semaphore.vi"("semaphore"=w228) -> ("error out"=w232:errorcluster, "semaphore out"=w230:T2)  [unwired: 4 in, 1 out]
                n115 = call "pumpStop.vi"("error in (no error)"=w232, "VISA resource name"=w226) -> ("error out"=w231:errorcluster)  [unwired: 9 in]
                n116 = call <vilib>:"Release Semaphore.vi"("error in (no error)"=w231, "semaphore"=w230) -> ()  [unwired: 4 in, 2 out]
              }
            }
          }
          event "HVEnable": Value Change {
            n117 = event-data() -> ("NewVal"=w233:bool)  [unwired: 1 in, 5 out]
            n118 = case shown="True" w233 {
              frame False {
                n119 = call "setDO.vi"("channel"=2, "on/off"=TRUE) -> ("错误输出"=w236:errorcluster)  [unwired: 9 in]
                n120 = call "setDO.vi"("错误输入（无错误）"=w236, "channel"=3, "on/off"=TRUE) -> ("错误输出"=w235:errorcluster)  [unwired: 8 in]
                n121 = call "setDO.vi"("错误输入（无错误）"=w235, "channel"=4, "on/off"=TRUE) -> ("错误输出"=w234:errorcluster)  [unwired: 8 in]
                n122 = call "setDO.vi"("错误输入（无错误）"=w234, "channel"=5, "on/off"=TRUE) -> ()  [unwired: 8 in, 1 out]
              }
              frame True {
                n123 = property on="MCPHV-Set" class="DigNum (strict)"() -> ("Value"=w269:dbl)  [unwired: 2 in, 2 out]
                n124 = Divide(x=w269, y=2000.0) -> (x/y=w271:dbl)
                n125 = Multiply(x=w271, y=10.0) -> (x*y=w262:dbl)
                n126 = Less?(x=w262, y=1.0) -> (x < y?=w263:bool)
                n127 = call "setDO.vi"("channel"=2, "on/off"=FALSE) -> ("错误输出"=w275:errorcluster)  [unwired: 9 in]
                n128 = case shown="False" w263 {
                  tunnel: w262 -> [w330 w338]
                  frame False {
                    n129 = while {
                      tunnel: w330 -> [w332]
                      tunnel: [w332] -> w328
                      i -> [w336]
                      stop <- w333 stop-if-true
                      n130 = Increment(x=w336) -> (x+1=w335:i32)
                      n131 = Increment(x=w335) -> (x+1=w334:i32)
                      n132 = call "setAO.vi"("value"=w335, "channel"=0) -> ()  [unwired: 9 in, 1 out]
                      n133 = Greater Or Equal?(x=w334, y=w332) -> (x >= y?=w333:bool)
                      n134 = Wait (ms)(milliseconds to wait=1000) -> ()  [unwired: 1 out]
                    }
                    n135 = call "setAO.vi"("value"=w328, "channel"=0) -> ()  [unwired: 9 in, 1 out]
                  }
                  frame True {
                    n136 = call "setAO.vi"("value"=w338, "channel"=0) -> ()  [unwired: 9 in, 1 out]
                  }
                }
                n137 = call "setDO.vi"("错误输入（无错误）"=w275, "channel"=3, "on/off"=FALSE) -> ("错误输出"=w274:errorcluster)  [unwired: 8 in]
                n138 = call "setDO.vi"("错误输入（无错误）"=w274, "channel"=4, "on/off"=FALSE) -> ("错误输出"=w273:errorcluster)  [unwired: 8 in]
                n139 = property on="Tar.HV-Set" class="DigNum (strict)"() -> ("Value"=w265:dbl)  [unwired: 2 in, 2 out]
                n140 = Divide(x=w265, y=20000.0) -> (x/y=w267:dbl)
                n141 = call "setDO.vi"("错误输入（无错误）"=w273, "channel"=5, "on/off"=FALSE) -> ()  [unwired: 8 in, 1 out]
                n142 = Multiply(x=w267, y=10.0) -> (x*y=w259:dbl)
                n143 = Less?(x=w259, y=0.5) -> (x < y?=w260:bool)
                n144 = case shown="False" w260 {
                  tunnel: w259 -> [w314 w326]
                  frame False {
                    n145 = while {
                      tunnel: w314 -> [w323]
                      tunnel: [w323] -> w312
                      i -> [w319]
                      stop <- w324 stop-if-true
                      n146 = Divide(x=w319, y=2.0) -> (x/y=w320:dbl)
                      n147 = Add(x=0.5, y=w320) -> (x+y=w317:dbl)
                      n148 = Add(x=w317, y=0.5) -> (x+y=w315:dbl)
                      n149 = call "setAO.vi"("value"=w317, "channel"=1) -> ()  [unwired: 9 in, 1 out]
                      n150 = Greater Or Equal?(x=w315, y=w323) -> (x >= y?=w324:bool)
                      n151 = Wait (ms)(milliseconds to wait=500) -> ()  [unwired: 1 out]
                    }
                    n152 = call "setAO.vi"("value"=w312, "channel"=1) -> ()  [unwired: 9 in, 1 out]
                  }
                  frame True {
                    n153 = call "setAO.vi"("value"=w326, "channel"=1) -> ()  [unwired: 9 in, 1 out]
                  }
                }
                n154 = property on="Pul.HV-Set" class="DigNum (strict)"() -> ("Value"=w258:dbl)  [unwired: 2 in, 2 out]
                n155 = Divide(x=w258, y=2000.0) -> (x/y=w253:dbl)
                n156 = Multiply(x=w253, y=10.0) -> (x*y=w257:dbl)
                n157 = Less?(x=w257, y=1.0) -> (x < y?=w256:bool)
                n158 = case shown="False" w256 {
                  tunnel: w257 -> [w302 w310]
                  frame False {
                    n159 = while {
                      tunnel: w302 -> [w304]
                      tunnel: [w304] -> w300
                      i -> [w308]
                      stop <- w305 stop-if-true
                      n160 = Increment(x=w308) -> (x+1=w307:i32)
                      n161 = Increment(x=w307) -> (x+1=w306:i32)
                      n162 = call "setAO.vi"("value"=w307, "channel"=2) -> ()  [unwired: 9 in, 1 out]
                      n163 = Greater Or Equal?(x=w306, y=w304) -> (x >= y?=w305:bool)
                      n164 = Wait (ms)(milliseconds to wait=1000) -> ()  [unwired: 1 out]
                    }
                    n165 = call "setAO.vi"("value"=w300, "channel"=2) -> ()  [unwired: 9 in, 1 out]
                  }
                  frame True {
                    n166 = call "setAO.vi"("value"=w310, "channel"=2) -> ()  [unwired: 9 in, 1 out]
                  }
                }
                n167 = property on="LensHV-Set" class="DigNum (strict)"() -> ("Value"=w251:dbl)  [unwired: 2 in, 2 out]
                n168 = Divide(x=w251, y=10000.0) -> (x/y=w246:dbl)
                n169 = Multiply(x=w246, y=10.0) -> (x*y=w250:dbl)
                n170 = Less?(x=w250, y=0.5) -> (x < y?=w249:bool)
                n171 = case shown="False" w249 {
                  tunnel: w250 -> [w286 w298]
                  frame False {
                    n172 = while {
                      tunnel: w286 -> [w295]
                      tunnel: [w295] -> w284
                      i -> [w291]
                      stop <- w296 stop-if-true
                      n173 = Divide(x=w291, y=2.0) -> (x/y=w292:dbl)
                      n174 = Add(x=0.5, y=w292) -> (x+y=w289:dbl)
                      n175 = Add(x=w289, y=0.5) -> (x+y=w287:dbl)
                      n176 = call "setAO.vi"("value"=w289, "channel"=3) -> ()  [unwired: 9 in, 1 out]
                      n177 = Greater Or Equal?(x=w287, y=w295) -> (x >= y?=w296:bool)
                      n178 = Wait (ms)(milliseconds to wait=500) -> ()  [unwired: 1 out]
                    }
                    n179 = call "setAO.vi"("value"=w284, "channel"=3) -> ()  [unwired: 9 in, 1 out]
                  }
                  frame True {
                    n180 = call "setAO.vi"("value"=w298, "channel"=3) -> ()  [unwired: 9 in, 1 out]
                  }
                }
              }
            }
          }
          event "Samp_Atmos": Value Change {
            n181 = event-data() -> ("OldVal"=w340:bool, "NewVal"=w344:bool)  [unwired: 1 in, 4 out]
            n182 = property on="Fore_Samp" class="Bool (strict)"() -> ("Value"=w343:bool)  [unwired: 2 in, 2 out]
            n183 = And(x=w344, y=w343) -> (x .and. y?=w342:bool)
            n184 = Not(x=w342) -> (.not. x?=w341:bool)
            n185 = case shown="True" w341 {
              tunnel: w344 -> [_ w347]
              tunnel: w340 -> [w346 _]
              frame False {
                n186 = property on="Samp_Atmos" class="Bool (strict)"("Value"=w346) -> (error out=w345:errorcluster)  [unwired: 2 in, 1 out]
                n187 = call "Display Message to User7"("error in (no error)"=w345) -> ()  [unwired: 9 in, 2 out]
              }
              frame True {
                n188 = case shown="False" w347 {
                  frame False {
                    n189 = call "setDO.vi"("channel"=6, "on/off"=FALSE) -> ()  [unwired: 9 in, 1 out]
                  }
                  frame True {
                    n190 = property on="Y满" class="Bool (strict)"() -> ("Value"=w351:bool)  [unwired: 2 in, 2 out]
                    n191 = Not(x=w351) -> (.not. x?=w350:bool)
                    n192 = case shown="False" w350 {
                      frame False {
                        n193 = call "setDO.vi"("channel"=6, "on/off"=TRUE) -> ()  [unwired: 9 in, 1 out]
                      }
                      frame True {
                        n194 = call "Display Message to User6"() -> ()  [unwired: 10 in, 2 out]
                      }
                    }
                  }
                }
              }
            }
          }
          event "Fore_Samp": Value Change {
            n195 = event-data() -> ("OldVal"=w354:bool, "NewVal"=w358:bool)  [unwired: 1 in, 4 out]
            n196 = property on="Samp_Atmos" class="Bool (strict)"() -> ("Value"=w357:bool)  [unwired: 2 in, 2 out]
            n197 = And(x=w358, y=w357) -> (x .and. y?=w356:bool)
            n198 = Not(x=w356) -> (.not. x?=w355:bool)
            n199 = case shown="True" w355 {
              tunnel: w358 -> [_ w361]
              tunnel: w354 -> [w360 _]
              frame False {
                n200 = property on="Fore_Samp" class="Bool (strict)"("Value"=w360) -> (error out=w359:errorcluster)  [unwired: 2 in, 1 out]
                n201 = call "Display Message to User8"("error in (no error)"=w359) -> ()  [unwired: 9 in, 2 out]
              }
              frame True {
                n202 = case shown="True" w361 {
                  frame False {
                    n203 = call "setDO.vi"("channel"=7, "on/off"=FALSE) -> ()  [unwired: 9 in, 1 out]
                  }
                  frame True {
                    n204 = property on="Y满" class="Bool (strict)"() -> ("Value"=w365:bool)  [unwired: 2 in, 2 out]
                    n205 = Not(x=w365) -> (.not. x?=w364:bool)
                    n206 = case shown="True" w364 {
                      frame False {
                        n207 = call "setDO.vi"("channel"=7, "on/off"=TRUE) -> ()  [unwired: 9 in, 1 out]
                      }
                      frame True {
                        n208 = call "Display Message to User"() -> ()  [unwired: 10 in, 2 out]
                      }
                    }
                  }
                }
              }
            }
          }
          event "MCPHV-Set": Value Change {
            n209 = event-data() -> ("NewVal"=w368:dbl)  [unwired: 1 in, 5 out]
            n210 = Divide(x=w368, y=2000.0) -> (x/y=w371:dbl)
            n211 = Multiply(x=w371, y=10.0) -> (x*y=w369:dbl)
            n212 = call "setAO.vi"("value"=w369, "channel"=0) -> ()  [unwired: 9 in, 1 out]
          }
          event "Tar.HV-Set": Value Change {
            n213 = event-data() -> ("NewVal"=w379:dbl)  [unwired: 1 in, 5 out]
            n214 = Divide(x=w379, y=20000.0) -> (x/y=w376:dbl)
            n215 = Multiply(x=w376, y=10.0) -> (x*y=w374:dbl)
            n216 = call "setAO.vi"("value"=w374, "channel"=1) -> ()  [unwired: 9 in, 1 out]
          }
          event "Pul.HV-Set": Value Change {
            n217 = event-data() -> ("NewVal"=w385:dbl)  [unwired: 1 in, 5 out]
            n218 = Divide(x=w385, y=2000.0) -> (x/y=w382:dbl)
            n219 = Multiply(x=w382, y=10.0) -> (x*y=w380:dbl)
            n220 = call "setAO.vi"("value"=w380, "channel"=2) -> ()  [unwired: 9 in, 1 out]
          }
          event "LensHV-Set": Value Change {
            n221 = event-data() -> ("NewVal"=w391:dbl)  [unwired: 1 in, 5 out]
            n222 = Divide(x=w391, y=10000.0) -> (x/y=w388:dbl)
            n223 = Multiply(x=w388, y=10.0) -> (x*y=w387:dbl)
            n224 = call "setAO.vi"("value"=w387, "channel"=3) -> ()  [unwired: 9 in, 1 out]
          }
          event User Event {
            n225 = event-data() -> ("status"=w392:string)  [unwired: 1 in, 5 out]
            n226 = case shown="\"stop\", Default" w392 {
              frame "stop", Default {
                n227 = property on="GO" class="Bool (strict)"("DisabledEnum"=T8."Enabled" ("Disabled")) -> (error out=w394:errorcluster)  [unwired: 2 in, 1 out]
                n228 = property on="移动" class="Bool (strict)"(error in=w394, "Value"=FALSE ("移动")) -> ()  [unwired: 1 in, 2 out]
              }
              frame "moving" {
                n229 = property on="GO" class="Bool (strict)"("DisabledEnum"=T8."Disabled and Grayed Out" ("Disabled")) -> (error out=w397:errorcluster)  [unwired: 2 in, 1 out]
                n230 = property on="移动" class="Bool (strict)"(error in=w397, "Value"=TRUE ("移动")) -> ()  [unwired: 1 in, 2 out]
              }
            }
          }
          event User Event {
            n231 = event-data() -> ("source"=w406:string, "value"=w405:dbl)  [unwired: 1 in, 4 out]
            n232 = case shown="\"X\"" w406 {
              tunnel: w405 -> [w407 w415]
              tunnel: [w409 w416] -> w399
              frame "Y", Default {
                n233 = property on="X当前" class="DigNum (strict)"() -> ("Value"=w411:dbl)  [unwired: 2 in, 2 out]
                n234 = Multiply(x=w407, y=1000.0) -> (x*y=w412:dbl)
                n235 = Divide(x=w411, y=1000.0) -> (x/y=w408:dbl)
                n236 = Build Array "Build Array"(w408, w407) -> (w409:dbl[])
                n237 = property on="Y当前" class="DigNum (strict)"("Value"=w412) -> ()  [unwired: 2 in, 2 out]
              }
              frame "X" {
                n238 = property on="Y当前" class="DigNum (strict)"() -> ("Value"=w418:dbl)  [unwired: 2 in, 2 out]
                n239 = Multiply(x=w415, y=1000.0) -> (x*y=w419:dbl)
                n240 = Divide(x=w418, y=1000.0) -> (x/y=w414:dbl)
                n241 = property on="X当前" class="DigNum (strict)"("Value"=w419) -> ()  [unwired: 2 in, 2 out]
                n242 = Build Array(w415, w414) -> (w416:dbl[])
              }
            }
            n243 = Current VI's Path() -> (path=w402:path)
            n244 = Strip Path(path=w402) -> (stripped path=w401:path)  [unwired: 1 out]
            n245 = Build Path(base path=w401, name or relative path="last_position") -> (appended path=w403:path)
            n246 = call-poly <vilib>:"Write To Spreadsheet File.vi"("format (%.3f)"="%.9f", "1D data"=w399, "file path (dialog if empty)"=w403) -> ()  [unwired: 5 in, 1 out]
          }
          event "TakeMS-Run": Value Change {
            n247 = event-data() -> ("NewVal"=w424:bool)  [unwired: 1 in, 5 out]
            n248 = case shown="True" w424 {
              tunnel: w423 -> [_ w437]
              tunnel: w422 -> [_ w434]
              tunnel: w421 -> [_ w433]
              frame False {
              }
              frame True {
                n249 = Unbundle By Name(w433) -> ("ConfiguredLaserCom"=w430:refnum<visa-resource-name>)
                n250 = Unbundle By Name(w434) -> ("laser semaphore"=w428:T2)
                n251 = property on="cluster" class="Clust (strict)"() -> ("Value"=w432:T6)  [unwired: 2 in, 2 out]
                n252 = Bundle By Name(cluster=w437, "ShotsPerPoint"="Shots/Point") -> (w435:T4)
                n253 = Unbundle By Name(w432) -> ("待机"=w429:bool)
                n254 = property on="SetLaserEnergy" class="Slide (strict)"() -> ("Value"=w427:dbl)  [unwired: 2 in, 2 out]
                n255 = Bundle By Name(cluster="Laser parameter", "VISA resource name"=w430, "standby"=w429, "semaphore in"=w428, "SetLaserEnergy"=w427) -> (w426:T3)
                n256 = case shown="0, Default" "AcquireMS-Methods" {
                  tunnel: w435 -> [w442 _ _]
                  tunnel: w426 -> [w443 _ _]
                  frame 0, Default {
                    n257 = call "Tiepie-takeData-2018-04-26.vi"("ADC parameter"=w442, "Laser parameter"=w443) -> ("output cluster"=w441:cluster{i32[], dbl[]})  [unwired: 2 in, 1 out]
                    "Mass Spectrum (质谱图)" <- w441
                    n258 = Unbundle(w441) -> (w440:i32[], w439:dbl[])
                    n259 = Build Array(w440, w439) -> (w438:dbl[][])
                    n260 = call-poly <vilib>:"Write To Spreadsheet File.vi"("2D data"=w438) -> ()  [unwired: 7 in, 1 out]
                  }
                  frame 1 {
                  }
                  frame 2 {
                  }
                }
              }
            }
          }
          event "Plat_To_Zero": Value Change {
            n261 = event-data() -> ("NewVal"=w444:bool)  [unwired: 1 in, 5 out]
            n262 = case shown="True" w444 {
              frame False {
              }
              frame True {
                n263 = call "plate_cal.vi"() -> ("错误输出"=w445:errorcluster)  [unwired: 11 in]
                n264 = property on="plat zeroed" class="Bool (strict)"(error in=w445, "Value"=TRUE ("plat zeroed")) -> ()  [unwired: 1 in, 2 out]
              }
            }
          }
          event "GO": Value Change {
            n265 = event-data() -> ("NewVal"=w448:bool)  [unwired: 1 in, 5 out]
            n266 = property on="移动" class="Bool (strict)"() -> ("Value"=w450:bool)  [unwired: 2 in, 2 out]
            n267 = Not(x=w450) -> (.not. x?=w449:bool)
            n268 = And(x=w449, y=w448) -> (x .and. y?=w447:bool)
            n269 = case shown="True" w447 {
              frame False {
              }
              frame True {
                n270 = property on="X" class="DigNum (strict)"() -> (error out=w455:errorcluster, "Value"=w453:dbl)  [unwired: 2 in, 1 out]
                n271 = property on="Y" class="DigNum (strict)"(error in=w455) -> (error out=w454:errorcluster, "Value"=w452:dbl)  [unwired: 1 in, 1 out]
                n272 = vi-ref "goto.vi"() -> (w459:refnum<vi>)
                n273 = property class="VI"(reference=w459, error in=w454) -> ("Name"=w458:string)  [unwired: 2 out]
                n274 = Open VI Reference(type specifier VI Refnum (for type only)=refnum<vi> refnum, vi path=w458, options=128) -> (vi reference=w456:refnum<vi>)  [unwired: 3 in, 1 out]
                n275 = call-by-ref "Start Asynchronous Call"(reference=w456, "Y(mm)"=w452, "X(mm)"=w453) -> ()  [unwired: 10 in, 3 out]
              }
            }
          }
          event "chamber in": Value Change {
            n276 = event-data() -> ("NewVal"=w461:bool)  [unwired: 1 in, 5 out]
            n277 = property on="HVEnable" class="Bool (strict)"() -> ("Value"=w466:bool)  [unwired: 2 in, 2 out]
            n278 = property on="Y满" class="Bool (strict)"() -> ("Value"=w462:bool)  [unwired: 2 in, 2 out]
            n279 = property on="移动" class="Bool (strict)"() -> ("Value"=w465:bool)  [unwired: 2 in, 2 out]
            n280 = Not(x=w466) -> (.not. x?=w463:bool)
            n281 = Not(x=w465) -> (.not. x?=w464:bool)
            n282 = Compound Arithmetic op=AND(w463, w462, w464, w461) -> (w460:bool)
            n283 = case shown="True" w460 {
              frame False {
              }
              frame True {
                n284 = flat-sequence {
                  tunnel: [w469] -> w467
                  tunnel: w467 -> [w478]
                  frame #0 {
                    w470 = FALSE ("on/off")
                    # "关样仓/大气"
                    n285 = Wait (ms)(milliseconds to wait=1500) -> ()  [unwired: 1 out]
                    n286 = call "setDO.vi"("channel"=6, "on/off"=w470) -> ("错误输出"=w468:errorcluster)  [unwired: 9 in]
                    n287 = property on="Samp_Atmos" class="Bool (strict)"(error in=w468, "Value"=w470) -> (error out=w469:errorcluster)  [unwired: 1 in, 1 out]
                  }
                  frame #1 {
                    # "开前泵/样仓"
                    n288 = call "setDO.vi"("错误输入（无错误）"=w478, "channel"=7, "on/off"=TRUE) -> ("错误输出"=w477:errorcluster)  [unwired: 8 in]
                    n289 = flat-sequence {
                      tunnel: w477 -> [w488]
                      tunnel: [w488] -> w473
                      frame #0 {
                        n290 = Wait (ms)(milliseconds to wait=10000) -> ()  [unwired: 1 out]
                      }
                    }
                    n291 = property on="Lvaccum" class="DigNum (strict)"() -> ("Value"=w476:dbl)  [unwired: 2 in, 2 out]
                    n292 = Less?(x=w476, y=1.0) -> (x < y?=w474:bool)
                    n293 = case shown="False" w474 {
                      tunnel: w473 -> [w482 w484]
                      frame False {
                        (unwired) 7
                        n294 = call "setDO.vi"("错误输入（无错误）"=w482, "on/off"=FALSE) -> ("错误输出"=w481:errorcluster)  [unwired: 9 in]
                        n295 = call "Display Message to User4"("error in (no error)"=w481) -> ()  [unwired: 9 in, 2 out]
                      }
                      frame True {
                        n296 = flat-sequence {
                          tunnel: w484 -> [w485]
                          frame #0 {
                            n297 = call "setDO.vi"("错误输入（无错误）"=w485, "channel"=7, "on/off"=FALSE) -> ()  [unwired: 8 in, 1 out]
                          }
                          frame #1 {
                            n298 = call "chamber_in.vi"() -> ()  [unwired: 12 in]
                          }
                        }
                      }
                    }
                  }
                }
              }
            }
          }
          event "chamber out": Value Change {
            n299 = event-data() -> ("NewVal"=w492:bool)  [unwired: 1 in, 5 out]
            n300 = property on="Y满" class="Bool (strict)"() -> ("Value"=w496:bool)  [unwired: 2 in, 2 out]
            n301 = property on="移动" class="Bool (strict)"() -> ("Value"=w495:bool)  [unwired: 2 in, 2 out]
            n302 = property on="HVEnable" class="Bool (strict)"() -> ("Value"=w497:bool)  [unwired: 2 in, 2 out]
            n303 = Not(x=w497) -> (.not. x?=w490:bool)
            n304 = Not(x=w495) -> (.not. x?=w493:bool)
            n305 = Not(x=w496) -> (.not. x?=w494:bool)
            n306 = Compound Arithmetic op=AND(w490, w494, w493, w492) -> (w491:bool)
            n307 = case shown="True" w491 {
              frame False {
                n308 = call "Display Message to User3"() -> ()  [unwired: 10 in, 2 out]
              }
              frame True {
                n309 = flat-sequence {
                  tunnel: [w501] -> w499
                  tunnel: w499 -> [w507]
                  tunnel: [w505] -> w498
                  tunnel: w498 -> [w516]
                  frame #0 {
                    n310 = call "chamber_out.vi"() -> ()  [unwired: 12 in]
                  }
                  frame #1 {
                    w502 = FALSE ("on/off")
                    # "关前泵/样仓"
                    n311 = Wait (ms)(milliseconds to wait=1500) -> ()  [unwired: 1 out]
                    n312 = call "setDO.vi"("channel"=7, "on/off"=w502) -> ("错误输出"=w500:errorcluster)  [unwired: 9 in]
                    n313 = property on="Fore_Samp" class="Bool (strict)"(error in=w500, "Value"=w502) -> (error out=w501:errorcluster)  [unwired: 1 in, 1 out]
                  }
                  frame #2 {
                    # "开样仓/大气"
                    n314 = property on="Y满" class="Bool (strict)"(error in=w507) -> (error out=w506:errorcluster, "Value"=w508:bool)  [unwired: 1 in, 1 out]
                    n315 = case shown="False" w508 {
                      tunnel: w506 -> [w511 w513]
                      tunnel: [w510 w512] -> w505
                      frame False {
                        n316 = call "Display Message to User2"("error in (no error)"=w511) -> ("error out"=w510:errorcluster)  [unwired: 9 in, 1 out]
                      }
                      frame True {
                        n317 = call "setDO.vi"("错误输入（无错误）"=w513, "channel"=6, "on/off"=TRUE) -> ("错误输出"=w512:errorcluster)  [unwired: 8 in]
                      }
                    }
                    n318 = Wait (ms)(milliseconds to wait=3000) -> ()  [unwired: 1 out]
                  }
                  frame #3 {
                    n319 = call "setDO.vi"("错误输入（无错误）"=w516, "channel"=6, "on/off"=FALSE) -> ()  [unwired: 8 in, 1 out]
                  }
                }
              }
            }
          }
          event "Image": Mouse Down {
            n320 = event-data() -> ("Coords"=w519:T13)  [unwired: 1 in, 7 out]
            n321 = property on="移动" class="Bool (strict)"() -> ("Value"=w520:bool)  [unwired: 2 in, 2 out]
            n322 = case shown="False" w520 {
              tunnel: w519 -> [w530 _]
              frame False {
                w527 = 0.01 ("x")
                n323 = Unbundle(w530) -> ("Horizontal"=w529:i32, "Vertical"=w528:i32)
                n324 = property on="X当前" class="DigNum (strict)"() -> ("Value"=w526:dbl)  [unwired: 2 in, 2 out]
                n325 = property on="Y当前" class="DigNum (strict)"() -> ("Value"=w522:dbl)  [unwired: 2 in, 2 out]
                n326 = Subtract(x=w529, y=222.0) -> (x-y=w532:dbl)
                n327 = Subtract(x=w528, y=201.0) -> (x-y=w531:dbl)
                n328 = Multiply(x=w527, y=w532) -> (x*y=w525:dbl)
                n329 = Multiply(x=w527, y=w531) -> (x*y=w523:dbl)
                n330 = Add(x=w526, y=w525) -> (x+y=w524:dbl)
                n331 = Add(x=w523, y=w522) -> (x+y=w521:dbl)
                n332 = call "goto.vi"("Y(mm)"=w521, "X(mm)"=w524) -> ()  [unwired: 9 in, 1 out]
              }
              frame True {
              }
            }
          }
          event "A1-Position": Value Change {
            n333 = event-data() -> ("NewVal"=w535:bool)  [unwired: 1 in, 5 out]
            n334 = case shown="True" w535 {
              frame False {
              }
              frame True {
                n335 = property on="X当前" class="DigNum (strict)"() -> ("Value"=→"A1-position-X":dbl)  [unwired: 2 in, 2 out]
                n336 = property on="Y当前" class="DigNum (strict)"() -> ("Value"=→"A1-position-Y":dbl)  [unwired: 2 in, 2 out]
              }
            }
          }
          event "A1": Value Change {
            n337 = event-data() -> ("NewVal"=w539:bool)  [unwired: 1 in, 5 out]
            n338 = property on="移动" class="Bool (strict)"() -> ("Value"=w541:bool)  [unwired: 2 in, 2 out]
            n339 = Not(x=w541) -> (.not. x?=w540:bool)
            n340 = And(x=w540, y=w539) -> (x .and. y?=w538:bool)
            n341 = case shown="True" w538 {
              frame False {
              }
              frame True {
                n342 = property on="A1-position-X" class="DigNum (strict)"() -> (error out=w546:errorcluster, "Value"=w544:dbl)  [unwired: 2 in, 1 out]
                n343 = property on="A1-position-Y" class="DigNum (strict)"(error in=w546) -> (error out=w545:errorcluster, "Value"=w543:dbl)  [unwired: 1 in, 1 out]
                n344 = vi-ref "goto.vi"() -> (w550:refnum<vi>)
                n345 = property class="VI"(reference=w550, error in=w545) -> ("Name"=w549:string)  [unwired: 2 out]
                n346 = Open VI Reference(type specifier VI Refnum (for type only)=refnum<vi> refnum, vi path=w549, options=128) -> (vi reference=w547:refnum<vi>)  [unwired: 3 in, 1 out]
                n347 = call-by-ref "Start Asynchronous Call"(reference=w547, "Y(mm)"=w543, "X(mm)"=w544) -> ()  [unwired: 10 in, 3 out]
              }
            }
          }
          event "A2": Value Change {
            n348 = event-data() -> ("NewVal"=w551:bool)  [unwired: 1 in, 5 out]
            n349 = property on="移动" class="Bool (strict)"() -> ("Value"=w554:bool)  [unwired: 2 in, 2 out]
            n350 = Not(x=w554) -> (.not. x?=w553:bool)
            n351 = And(x=w553, y=w551) -> (x .and. y?=w552:bool)
            n352 = case shown="True" w552 {
              frame False {
              }
              frame True {
                n353 = property on="A1-position-X" class="DigNum (strict)"() -> (error out=w558:errorcluster, "Value"=w565:dbl)  [unwired: 2 in, 1 out]
                n354 = property on="A1-position-Y" class="DigNum (strict)"(error in=w558) -> (error out=w557:errorcluster, "Value"=w555:dbl)  [unwired: 1 in, 1 out]
                n355 = Subtract(x=w565, y=4.5) -> (x-y=w556:dbl)
                n356 = vi-ref "goto.vi"() -> (w563:refnum<vi>)
                n357 = property class="VI"(reference=w563, error in=w557) -> ("Name"=w562:string)  [unwired: 2 out]
                n358 = Open VI Reference(type specifier VI Refnum (for type only)=refnum<vi> refnum, vi path=w562, options=128) -> (vi reference=w560:refnum<vi>)  [unwired: 3 in, 1 out]
                n359 = call-by-ref "Start Asynchronous Call"(reference=w560, "Y(mm)"=w555, "X(mm)"=w556) -> ()  [unwired: 10 in, 3 out]
              }
            }
          }
          event "A3": Value Change {
            n360 = event-data() -> ("NewVal"=w566:bool)  [unwired: 1 in, 5 out]
            n361 = property on="移动" class="Bool (strict)"() -> ("Value"=w569:bool)  [unwired: 2 in, 2 out]
            n362 = Not(x=w569) -> (.not. x?=w568:bool)
            n363 = And(x=w568, y=w566) -> (x .and. y?=w567:bool)
            n364 = case shown="True" w567 {
              frame False {
              }
              frame True {
                n365 = property on="A1-position-X" class="DigNum (strict)"() -> (error out=w573:errorcluster, "Value"=w580:dbl)  [unwired: 2 in, 1 out]
                n366 = property on="A1-position-Y" class="DigNum (strict)"(error in=w573) -> (error out=w572:errorcluster, "Value"=w570:dbl)  [unwired: 1 in, 1 out]
                n367 = Subtract(x=w580, y=9.0) -> (x-y=w571:dbl)
                n368 = vi-ref "goto.vi"() -> (w578:refnum<vi>)
                n369 = property class="VI"(reference=w578, error in=w572) -> ("Name"=w577:string)  [unwired: 2 out]
                n370 = Open VI Reference(type specifier VI Refnum (for type only)=refnum<vi> refnum, vi path=w577, options=128) -> (vi reference=w575:refnum<vi>)  [unwired: 3 in, 1 out]
                n371 = call-by-ref "Start Asynchronous Call"(reference=w575, "Y(mm)"=w570, "X(mm)"=w571) -> ()  [unwired: 10 in, 3 out]
              }
            }
          }
          event "A4": Value Change {
            n372 = event-data() -> ("NewVal"=w581:bool)  [unwired: 1 in, 5 out]
            n373 = property on="移动" class="Bool (strict)"() -> ("Value"=w584:bool)  [unwired: 2 in, 2 out]
            n374 = Not(x=w584) -> (.not. x?=w583:bool)
            n375 = And(x=w583, y=w581) -> (x .and. y?=w582:bool)
            n376 = case shown="True" w582 {
              frame False {
              }
              frame True {
                n377 = property on="A1-position-X" class="DigNum (strict)"() -> (error out=w588:errorcluster, "Value"=w595:dbl)  [unwired: 2 in, 1 out]
                n378 = property on="A1-position-Y" class="DigNum (strict)"(error in=w588) -> (error out=w587:errorcluster, "Value"=w585:dbl)  [unwired: 1 in, 1 out]
                n379 = Subtract(x=w595, y=13.5) -> (x-y=w586:dbl)
                n380 = vi-ref "goto.vi"() -> (w593:refnum<vi>)
                n381 = property class="VI"(reference=w593, error in=w587) -> ("Name"=w592:string)  [unwired: 2 out]
                n382 = Open VI Reference(type specifier VI Refnum (for type only)=refnum<vi> refnum, vi path=w592, options=128) -> (vi reference=w590:refnum<vi>)  [unwired: 3 in, 1 out]
                n383 = call-by-ref "Start Asynchronous Call"(reference=w590, "Y(mm)"=w585, "X(mm)"=w586) -> ()  [unwired: 10 in, 3 out]
              }
            }
          }
          event "A5": Value Change {
            n384 = event-data() -> ("NewVal"=w596:bool)  [unwired: 1 in, 5 out]
            n385 = property on="移动" class="Bool (strict)"() -> ("Value"=w599:bool)  [unwired: 2 in, 2 out]
            n386 = Not(x=w599) -> (.not. x?=w598:bool)
            n387 = And(x=w598, y=w596) -> (x .and. y?=w597:bool)
            n388 = case shown="True" w597 {
              frame False {
              }
              frame True {
                n389 = property on="A1-position-X" class="DigNum (strict)"() -> (error out=w603:errorcluster, "Value"=w610:dbl)  [unwired: 2 in, 1 out]
                n390 = property on="A1-position-Y" class="DigNum (strict)"(error in=w603) -> (error out=w602:errorcluster, "Value"=w600:dbl)  [unwired: 1 in, 1 out]
                n391 = Subtract(x=w610, y=18) -> (x-y=w601:dbl)
                n392 = vi-ref "goto.vi"() -> (w608:refnum<vi>)
                n393 = property class="VI"(reference=w608, error in=w602) -> ("Name"=w607:string)  [unwired: 2 out]
                n394 = Open VI Reference(type specifier VI Refnum (for type only)=refnum<vi> refnum, vi path=w607, options=128) -> (vi reference=w605:refnum<vi>)  [unwired: 3 in, 1 out]
                n395 = call-by-ref "Start Asynchronous Call"(reference=w605, "Y(mm)"=w600, "X(mm)"=w601) -> ()  [unwired: 10 in, 3 out]
              }
            }
          }
          event "A6": Value Change {
            n396 = event-data() -> ("NewVal"=w611:bool)  [unwired: 1 in, 5 out]
            n397 = property on="移动" class="Bool (strict)"() -> ("Value"=w614:bool)  [unwired: 2 in, 2 out]
            n398 = Not(x=w614) -> (.not. x?=w613:bool)
            n399 = And(x=w613, y=w611) -> (x .and. y?=w612:bool)
            n400 = case shown="True" w612 {
              frame False {
              }
              frame True {
                n401 = property on="A1-position-X" class="DigNum (strict)"() -> (error out=w618:errorcluster, "Value"=w625:dbl)  [unwired: 2 in, 1 out]
                n402 = property on="A1-position-Y" class="DigNum (strict)"(error in=w618) -> (error out=w617:errorcluster, "Value"=w615:dbl)  [unwired: 1 in, 1 out]
                n403 = Subtract(x=w625, y=22.5) -> (x-y=w616:dbl)
                n404 = vi-ref "goto.vi"() -> (w623:refnum<vi>)
                n405 = property class="VI"(reference=w623, error in=w617) -> ("Name"=w622:string)  [unwired: 2 out]
                n406 = Open VI Reference(type specifier VI Refnum (for type only)=refnum<vi> refnum, vi path=w622, options=128) -> (vi reference=w620:refnum<vi>)  [unwired: 3 in, 1 out]
                n407 = call-by-ref "Start Asynchronous Call"(reference=w620, "Y(mm)"=w615, "X(mm)"=w616) -> ()  [unwired: 10 in, 3 out]
              }
            }
          }
          event "A7": Value Change {
            n408 = event-data() -> ("NewVal"=w626:bool)  [unwired: 1 in, 5 out]
            n409 = property on="移动" class="Bool (strict)"() -> ("Value"=w629:bool)  [unwired: 2 in, 2 out]
            n410 = Not(x=w629) -> (.not. x?=w628:bool)
            n411 = And(x=w628, y=w626) -> (x .and. y?=w627:bool)
            n412 = case shown="True" w627 {
              frame False {
              }
              frame True {
                n413 = property on="A1-position-X" class="DigNum (strict)"() -> (error out=w633:errorcluster, "Value"=w640:dbl)  [unwired: 2 in, 1 out]
                n414 = property on="A1-position-Y" class="DigNum (strict)"(error in=w633) -> (error out=w632:errorcluster, "Value"=w630:dbl)  [unwired: 1 in, 1 out]
                n415 = Subtract(x=w640, y=27) -> (x-y=w631:dbl)
                n416 = vi-ref "goto.vi"() -> (w638:refnum<vi>)
                n417 = property class="VI"(reference=w638, error in=w632) -> ("Name"=w637:string)  [unwired: 2 out]
                n418 = Open VI Reference(type specifier VI Refnum (for type only)=refnum<vi> refnum, vi path=w637, options=128) -> (vi reference=w635:refnum<vi>)  [unwired: 3 in, 1 out]
                n419 = call-by-ref "Start Asynchronous Call"(reference=w635, "Y(mm)"=w630, "X(mm)"=w631) -> ()  [unwired: 10 in, 3 out]
              }
            }
          }
          event "A8": Value Change {
            n420 = event-data() -> ("NewVal"=w641:bool)  [unwired: 1 in, 5 out]
            n421 = property on="移动" class="Bool (strict)"() -> ("Value"=w644:bool)  [unwired: 2 in, 2 out]
            n422 = Not(x=w644) -> (.not. x?=w643:bool)
            n423 = And(x=w643, y=w641) -> (x .and. y?=w642:bool)
            n424 = case shown="True" w642 {
              frame False {
              }
              frame True {
                n425 = property on="A1-position-X" class="DigNum (strict)"() -> (error out=w648:errorcluster, "Value"=w655:dbl)  [unwired: 2 in, 1 out]
                n426 = property on="A1-position-Y" class="DigNum (strict)"(error in=w648) -> (error out=w647:errorcluster, "Value"=w645:dbl)  [unwired: 1 in, 1 out]
                n427 = Subtract(x=w655, y=31.5) -> (x-y=w646:dbl)
                n428 = vi-ref "goto.vi"() -> (w653:refnum<vi>)
                n429 = property class="VI"(reference=w653, error in=w647) -> ("Name"=w652:string)  [unwired: 2 out]
                n430 = Open VI Reference(type specifier VI Refnum (for type only)=refnum<vi> refnum, vi path=w652, options=128) -> (vi reference=w650:refnum<vi>)  [unwired: 3 in, 1 out]
                n431 = call-by-ref "Start Asynchronous Call"(reference=w650, "Y(mm)"=w645, "X(mm)"=w646) -> ()  [unwired: 10 in, 3 out]
              }
            }
          }
          event "A9": Value Change {
            n432 = event-data() -> ("NewVal"=w656:bool)  [unwired: 1 in, 5 out]
            n433 = property on="移动" class="Bool (strict)"() -> ("Value"=w659:bool)  [unwired: 2 in, 2 out]
            n434 = Not(x=w659) -> (.not. x?=w658:bool)
            n435 = And(x=w658, y=w656) -> (x .and. y?=w657:bool)
            n436 = case shown="True" w657 {
              frame False {
              }
              frame True {
                n437 = property on="A1-position-X" class="DigNum (strict)"() -> (error out=w663:errorcluster, "Value"=w670:dbl)  [unwired: 2 in, 1 out]
                n438 = property on="A1-position-Y" class="DigNum (strict)"(error in=w663) -> (error out=w662:errorcluster, "Value"=w660:dbl)  [unwired: 1 in, 1 out]
                n439 = Subtract(x=w670, y=36) -> (x-y=w661:dbl)
                n440 = vi-ref "goto.vi"() -> (w668:refnum<vi>)
                n441 = property class="VI"(reference=w668, error in=w662) -> ("Name"=w667:string)  [unwired: 2 out]
                n442 = Open VI Reference(type specifier VI Refnum (for type only)=refnum<vi> refnum, vi path=w667, options=128) -> (vi reference=w665:refnum<vi>)  [unwired: 3 in, 1 out]
                n443 = call-by-ref "Start Asynchronous Call"(reference=w665, "Y(mm)"=w660, "X(mm)"=w661) -> ()  [unwired: 10 in, 3 out]
              }
            }
          }
          event "A10": Value Change {
            n444 = event-data() -> ("NewVal"=w671:bool)  [unwired: 1 in, 5 out]
            n445 = property on="移动" class="Bool (strict)"() -> ("Value"=w674:bool)  [unwired: 2 in, 2 out]
            n446 = Not(x=w674) -> (.not. x?=w673:bool)
            n447 = And(x=w673, y=w671) -> (x .and. y?=w672:bool)
            n448 = case shown="True" w672 {
              frame False {
              }
              frame True {
                n449 = property on="A1-position-X" class="DigNum (strict)"() -> (error out=w678:errorcluster, "Value"=w685:dbl)  [unwired: 2 in, 1 out]
                n450 = property on="A1-position-Y" class="DigNum (strict)"(error in=w678) -> (error out=w677:errorcluster, "Value"=w675:dbl)  [unwired: 1 in, 1 out]
                n451 = Subtract(x=w685, y=40.5) -> (x-y=w676:dbl)
                n452 = vi-ref "goto.vi"() -> (w683:refnum<vi>)
                n453 = property class="VI"(reference=w683, error in=w677) -> ("Name"=w682:string)  [unwired: 2 out]
                n454 = Open VI Reference(type specifier VI Refnum (for type only)=refnum<vi> refnum, vi path=w682, options=128) -> (vi reference=w680:refnum<vi>)  [unwired: 3 in, 1 out]
                n455 = call-by-ref "Start Asynchronous Call"(reference=w680, "Y(mm)"=w675, "X(mm)"=w676) -> ()  [unwired: 10 in, 3 out]
              }
            }
          }
          event "A11": Value Change {
            n456 = event-data() -> ("NewVal"=w686:bool)  [unwired: 1 in, 5 out]
            n457 = property on="移动" class="Bool (strict)"() -> ("Value"=w689:bool)  [unwired: 2 in, 2 out]
            n458 = Not(x=w689) -> (.not. x?=w688:bool)
            n459 = And(x=w688, y=w686) -> (x .and. y?=w687:bool)
            n460 = case shown="True" w687 {
              frame False {
              }
              frame True {
                n461 = property on="A1-position-X" class="DigNum (strict)"() -> (error out=w693:errorcluster, "Value"=w700:dbl)  [unwired: 2 in, 1 out]
                n462 = property on="A1-position-Y" class="DigNum (strict)"(error in=w693) -> (error out=w692:errorcluster, "Value"=w690:dbl)  [unwired: 1 in, 1 out]
                n463 = Subtract(x=w700, y=45) -> (x-y=w691:dbl)
                n464 = vi-ref "goto.vi"() -> (w698:refnum<vi>)
                n465 = property class="VI"(reference=w698, error in=w692) -> ("Name"=w697:string)  [unwired: 2 out]
                n466 = Open VI Reference(type specifier VI Refnum (for type only)=refnum<vi> refnum, vi path=w697, options=128) -> (vi reference=w695:refnum<vi>)  [unwired: 3 in, 1 out]
                n467 = call-by-ref "Start Asynchronous Call"(reference=w695, "Y(mm)"=w690, "X(mm)"=w691) -> ()  [unwired: 10 in, 3 out]
              }
            }
          }
          event "A12": Value Change {
            n468 = event-data() -> ("NewVal"=w701:bool)  [unwired: 1 in, 5 out]
            n469 = property on="移动" class="Bool (strict)"() -> ("Value"=w704:bool)  [unwired: 2 in, 2 out]
            n470 = Not(x=w704) -> (.not. x?=w703:bool)
            n471 = And(x=w703, y=w701) -> (x .and. y?=w702:bool)
            n472 = case shown="True" w702 {
              frame False {
              }
              frame True {
                n473 = property on="A1-position-X" class="DigNum (strict)"() -> (error out=w708:errorcluster, "Value"=w715:dbl)  [unwired: 2 in, 1 out]
                n474 = property on="A1-position-Y" class="DigNum (strict)"(error in=w708) -> (error out=w707:errorcluster, "Value"=w705:dbl)  [unwired: 1 in, 1 out]
                n475 = Subtract(x=w715, y=49.5) -> (x-y=w706:dbl)
                n476 = vi-ref "goto.vi"() -> (w713:refnum<vi>)
                n477 = property class="VI"(reference=w713, error in=w707) -> ("Name"=w712:string)  [unwired: 2 out]
                n478 = Open VI Reference(type specifier VI Refnum (for type only)=refnum<vi> refnum, vi path=w712, options=128) -> (vi reference=w710:refnum<vi>)  [unwired: 3 in, 1 out]
                n479 = call-by-ref "Start Asynchronous Call"(reference=w710, "Y(mm)"=w705, "X(mm)"=w706) -> ()  [unwired: 10 in, 3 out]
              }
            }
          }
          event "B1": Value Change {
            n480 = event-data() -> ("NewVal"=w716:bool)  [unwired: 1 in, 5 out]
            n481 = property on="移动" class="Bool (strict)"() -> ("Value"=w719:bool)  [unwired: 2 in, 2 out]
            n482 = Not(x=w719) -> (.not. x?=w718:bool)
            n483 = And(x=w718, y=w716) -> (x .and. y?=w717:bool)
            n484 = case shown="True" w717 {
              frame False {
              }
              frame True {
                n485 = property on="A1-position-X" class="DigNum (strict)"() -> (error out=w725:errorcluster, "Value"=w732:dbl)  [unwired: 2 in, 1 out]
                n486 = property on="A1-position-Y" class="DigNum (strict)"(error in=w725) -> (error out=w724:errorcluster, "Value"=w721:dbl)  [unwired: 1 in, 1 out]
                n487 = Subtract(x=w721, y=4.5) -> (x-y=w720:dbl)
                n488 = Subtract(x=w732, y=0) -> (x-y=w723:dbl)
                n489 = vi-ref "goto.vi"() -> (w730:refnum<vi>)
                n490 = property class="VI"(reference=w730, error in=w724) -> ("Name"=w729:string)  [unwired: 2 out]
                n491 = Open VI Reference(type specifier VI Refnum (for type only)=refnum<vi> refnum, vi path=w729, options=128) -> (vi reference=w727:refnum<vi>)  [unwired: 3 in, 1 out]
                n492 = call-by-ref "Start Asynchronous Call"(reference=w727, "Y(mm)"=w720, "X(mm)"=w723) -> ()  [unwired: 10 in, 3 out]
              }
            }
          }
          event "B2": Value Change {
            n493 = event-data() -> ("NewVal"=w733:bool)  [unwired: 1 in, 5 out]
            n494 = property on="移动" class="Bool (strict)"() -> ("Value"=w736:bool)  [unwired: 2 in, 2 out]
            n495 = Not(x=w736) -> (.not. x?=w735:bool)
            n496 = And(x=w735, y=w733) -> (x .and. y?=w734:bool)
            n497 = case shown="True" w734 {
              frame False {
              }
              frame True {
                n498 = property on="A1-position-X" class="DigNum (strict)"() -> (error out=w742:errorcluster, "Value"=w749:dbl)  [unwired: 2 in, 1 out]
                n499 = property on="A1-position-Y" class="DigNum (strict)"(error in=w742) -> (error out=w741:errorcluster, "Value"=w738:dbl)  [unwired: 1 in, 1 out]
                n500 = Subtract(x=w738, y=4.5) -> (x-y=w737:dbl)
                n501 = Subtract(x=w749, y=4.5) -> (x-y=w740:dbl)
                n502 = vi-ref "goto.vi"() -> (w747:refnum<vi>)
                n503 = property class="VI"(reference=w747, error in=w741) -> ("Name"=w746:string)  [unwired: 2 out]
                n504 = Open VI Reference(type specifier VI Refnum (for type only)=refnum<vi> refnum, vi path=w746, options=128) -> (vi reference=w744:refnum<vi>)  [unwired: 3 in, 1 out]
                n505 = call-by-ref "Start Asynchronous Call"(reference=w744, "Y(mm)"=w737, "X(mm)"=w740) -> ()  [unwired: 10 in, 3 out]
              }
            }
          }
          event "B3": Value Change {
            n506 = event-data() -> ("NewVal"=w750:bool)  [unwired: 1 in, 5 out]
            n507 = property on="移动" class="Bool (strict)"() -> ("Value"=w753:bool)  [unwired: 2 in, 2 out]
            n508 = Not(x=w753) -> (.not. x?=w752:bool)
            n509 = And(x=w752, y=w750) -> (x .and. y?=w751:bool)
            n510 = case shown="True" w751 {
              frame False {
              }
              frame True {
                n511 = property on="A1-position-X" class="DigNum (strict)"() -> (error out=w759:errorcluster, "Value"=w766:dbl)  [unwired: 2 in, 1 out]
                n512 = property on="A1-position-Y" class="DigNum (strict)"(error in=w759) -> (error out=w758:errorcluster, "Value"=w755:dbl)  [unwired: 1 in, 1 out]
                n513 = Subtract(x=w755, y=4.5) -> (x-y=w754:dbl)
                n514 = Subtract(x=w766, y=9) -> (x-y=w757:dbl)
                n515 = vi-ref "goto.vi"() -> (w764:refnum<vi>)
                n516 = property class="VI"(reference=w764, error in=w758) -> ("Name"=w763:string)  [unwired: 2 out]
                n517 = Open VI Reference(type specifier VI Refnum (for type only)=refnum<vi> refnum, vi path=w763, options=128) -> (vi reference=w761:refnum<vi>)  [unwired: 3 in, 1 out]
                n518 = call-by-ref "Start Asynchronous Call"(reference=w761, "Y(mm)"=w754, "X(mm)"=w757) -> ()  [unwired: 10 in, 3 out]
              }
            }
          }
          event "B4": Value Change {
            n519 = event-data() -> ("NewVal"=w767:bool)  [unwired: 1 in, 5 out]
            n520 = property on="移动" class="Bool (strict)"() -> ("Value"=w770:bool)  [unwired: 2 in, 2 out]
            n521 = Not(x=w770) -> (.not. x?=w769:bool)
            n522 = And(x=w769, y=w767) -> (x .and. y?=w768:bool)
            n523 = case shown="True" w768 {
              frame False {
              }
              frame True {
                n524 = property on="A1-position-X" class="DigNum (strict)"() -> (error out=w776:errorcluster, "Value"=w783:dbl)  [unwired: 2 in, 1 out]
                n525 = property on="A1-position-Y" class="DigNum (strict)"(error in=w776) -> (error out=w775:errorcluster, "Value"=w772:dbl)  [unwired: 1 in, 1 out]
                n526 = Subtract(x=w772, y=4.5) -> (x-y=w771:dbl)
                n527 = Subtract(x=w783, y=13.5) -> (x-y=w774:dbl)
                n528 = vi-ref "goto.vi"() -> (w781:refnum<vi>)
                n529 = property class="VI"(reference=w781, error in=w775) -> ("Name"=w780:string)  [unwired: 2 out]
                n530 = Open VI Reference(type specifier VI Refnum (for type only)=refnum<vi> refnum, vi path=w780, options=128) -> (vi reference=w778:refnum<vi>)  [unwired: 3 in, 1 out]
                n531 = call-by-ref "Start Asynchronous Call"(reference=w778, "Y(mm)"=w771, "X(mm)"=w774) -> ()  [unwired: 10 in, 3 out]
              }
            }
          }
          event "B5": Value Change {
            n532 = event-data() -> ("NewVal"=w784:bool)  [unwired: 1 in, 5 out]
            n533 = property on="移动" class="Bool (strict)"() -> ("Value"=w787:bool)  [unwired: 2 in, 2 out]
            n534 = Not(x=w787) -> (.not. x?=w786:bool)
            n535 = And(x=w786, y=w784) -> (x .and. y?=w785:bool)
            n536 = case shown="True" w785 {
              frame False {
              }
              frame True {
                n537 = property on="A1-position-X" class="DigNum (strict)"() -> (error out=w793:errorcluster, "Value"=w800:dbl)  [unwired: 2 in, 1 out]
                n538 = property on="A1-position-Y" class="DigNum (strict)"(error in=w793) -> (error out=w792:errorcluster, "Value"=w789:dbl)  [unwired: 1 in, 1 out]
                n539 = Subtract(x=w789, y=4.5) -> (x-y=w788:dbl)
                n540 = Subtract(x=w800, y=18) -> (x-y=w791:dbl)
                n541 = vi-ref "goto.vi"() -> (w798:refnum<vi>)
                n542 = property class="VI"(reference=w798, error in=w792) -> ("Name"=w797:string)  [unwired: 2 out]
                n543 = Open VI Reference(type specifier VI Refnum (for type only)=refnum<vi> refnum, vi path=w797, options=128) -> (vi reference=w795:refnum<vi>)  [unwired: 3 in, 1 out]
                n544 = call-by-ref "Start Asynchronous Call"(reference=w795, "Y(mm)"=w788, "X(mm)"=w791) -> ()  [unwired: 10 in, 3 out]
              }
            }
          }
          event "B6": Value Change {
            n545 = event-data() -> ("NewVal"=w801:bool)  [unwired: 1 in, 5 out]
            n546 = property on="移动" class="Bool (strict)"() -> ("Value"=w804:bool)  [unwired: 2 in, 2 out]
            n547 = Not(x=w804) -> (.not. x?=w803:bool)
            n548 = And(x=w803, y=w801) -> (x .and. y?=w802:bool)
            n549 = case shown="True" w802 {
              frame False {
              }
              frame True {
                n550 = property on="A1-position-X" class="DigNum (strict)"() -> (error out=w810:errorcluster, "Value"=w817:dbl)  [unwired: 2 in, 1 out]
                n551 = property on="A1-position-Y" class="DigNum (strict)"(error in=w810) -> (error out=w809:errorcluster, "Value"=w806:dbl)  [unwired: 1 in, 1 out]
                n552 = Subtract(x=w806, y=4.5) -> (x-y=w805:dbl)
                n553 = Subtract(x=w817, y=22.5) -> (x-y=w808:dbl)
                n554 = vi-ref "goto.vi"() -> (w815:refnum<vi>)
                n555 = property class="VI"(reference=w815, error in=w809) -> ("Name"=w814:string)  [unwired: 2 out]
                n556 = Open VI Reference(type specifier VI Refnum (for type only)=refnum<vi> refnum, vi path=w814, options=128) -> (vi reference=w812:refnum<vi>)  [unwired: 3 in, 1 out]
                n557 = call-by-ref "Start Asynchronous Call"(reference=w812, "Y(mm)"=w805, "X(mm)"=w808) -> ()  [unwired: 10 in, 3 out]
              }
            }
          }
          event "B7": Value Change {
            n558 = event-data() -> ("NewVal"=w818:bool)  [unwired: 1 in, 5 out]
            n559 = property on="移动" class="Bool (strict)"() -> ("Value"=w821:bool)  [unwired: 2 in, 2 out]
            n560 = Not(x=w821) -> (.not. x?=w820:bool)
            n561 = And(x=w820, y=w818) -> (x .and. y?=w819:bool)
            n562 = case shown="True" w819 {
              frame False {
              }
              frame True {
                n563 = property on="A1-position-X" class="DigNum (strict)"() -> (error out=w827:errorcluster, "Value"=w834:dbl)  [unwired: 2 in, 1 out]
                n564 = property on="A1-position-Y" class="DigNum (strict)"(error in=w827) -> (error out=w826:errorcluster, "Value"=w823:dbl)  [unwired: 1 in, 1 out]
                n565 = Subtract(x=w823, y=4.5) -> (x-y=w822:dbl)
                n566 = Subtract(x=w834, y=27) -> (x-y=w825:dbl)
                n567 = vi-ref "goto.vi"() -> (w832:refnum<vi>)
                n568 = property class="VI"(reference=w832, error in=w826) -> ("Name"=w831:string)  [unwired: 2 out]
                n569 = Open VI Reference(type specifier VI Refnum (for type only)=refnum<vi> refnum, vi path=w831, options=128) -> (vi reference=w829:refnum<vi>)  [unwired: 3 in, 1 out]
                n570 = call-by-ref "Start Asynchronous Call"(reference=w829, "Y(mm)"=w822, "X(mm)"=w825) -> ()  [unwired: 10 in, 3 out]
              }
            }
          }
          event "B8": Value Change {
            n571 = event-data() -> ("NewVal"=w835:bool)  [unwired: 1 in, 5 out]
            n572 = property on="移动" class="Bool (strict)"() -> ("Value"=w838:bool)  [unwired: 2 in, 2 out]
            n573 = Not(x=w838) -> (.not. x?=w837:bool)
            n574 = And(x=w837, y=w835) -> (x .and. y?=w836:bool)
            n575 = case shown="True" w836 {
              frame False {
              }
              frame True {
                n576 = property on="A1-position-X" class="DigNum (strict)"() -> (error out=w844:errorcluster, "Value"=w851:dbl)  [unwired: 2 in, 1 out]
                n577 = property on="A1-position-Y" class="DigNum (strict)"(error in=w844) -> (error out=w843:errorcluster, "Value"=w840:dbl)  [unwired: 1 in, 1 out]
                n578 = Subtract(x=w840, y=4.5) -> (x-y=w839:dbl)
                n579 = Subtract(x=w851, y=31.5) -> (x-y=w842:dbl)
                n580 = vi-ref "goto.vi"() -> (w849:refnum<vi>)
                n581 = property class="VI"(reference=w849, error in=w843) -> ("Name"=w848:string)  [unwired: 2 out]
                n582 = Open VI Reference(type specifier VI Refnum (for type only)=refnum<vi> refnum, vi path=w848, options=128) -> (vi reference=w846:refnum<vi>)  [unwired: 3 in, 1 out]
                n583 = call-by-ref "Start Asynchronous Call"(reference=w846, "Y(mm)"=w839, "X(mm)"=w842) -> ()  [unwired: 10 in, 3 out]
              }
            }
          }
          event "B9": Value Change {
            n584 = event-data() -> ("NewVal"=w852:bool)  [unwired: 1 in, 5 out]
            n585 = property on="移动" class="Bool (strict)"() -> ("Value"=w855:bool)  [unwired: 2 in, 2 out]
            n586 = Not(x=w855) -> (.not. x?=w854:bool)
            n587 = And(x=w854, y=w852) -> (x .and. y?=w853:bool)
            n588 = case shown="True" w853 {
              frame False {
              }
              frame True {
                n589 = property on="A1-position-X" class="DigNum (strict)"() -> (error out=w861:errorcluster, "Value"=w868:dbl)  [unwired: 2 in, 1 out]
                n590 = property on="A1-position-Y" class="DigNum (strict)"(error in=w861) -> (error out=w860:errorcluster, "Value"=w857:dbl)  [unwired: 1 in, 1 out]
                n591 = Subtract(x=w857, y=4.5) -> (x-y=w856:dbl)
                n592 = Subtract(x=w868, y=36) -> (x-y=w859:dbl)
                n593 = vi-ref "goto.vi"() -> (w866:refnum<vi>)
                n594 = property class="VI"(reference=w866, error in=w860) -> ("Name"=w865:string)  [unwired: 2 out]
                n595 = Open VI Reference(type specifier VI Refnum (for type only)=refnum<vi> refnum, vi path=w865, options=128) -> (vi reference=w863:refnum<vi>)  [unwired: 3 in, 1 out]
                n596 = call-by-ref "Start Asynchronous Call"(reference=w863, "Y(mm)"=w856, "X(mm)"=w859) -> ()  [unwired: 10 in, 3 out]
              }
            }
          }
          event "B10": Value Change {
            n597 = event-data() -> ("NewVal"=w869:bool)  [unwired: 1 in, 5 out]
            n598 = property on="移动" class="Bool (strict)"() -> ("Value"=w872:bool)  [unwired: 2 in, 2 out]
            n599 = Not(x=w872) -> (.not. x?=w871:bool)
            n600 = And(x=w871, y=w869) -> (x .and. y?=w870:bool)
            n601 = case shown="True" w870 {
              frame False {
              }
              frame True {
                n602 = property on="A1-position-X" class="DigNum (strict)"() -> (error out=w878:errorcluster, "Value"=w885:dbl)  [unwired: 2 in, 1 out]
                n603 = property on="A1-position-Y" class="DigNum (strict)"(error in=w878) -> (error out=w877:errorcluster, "Value"=w874:dbl)  [unwired: 1 in, 1 out]
                n604 = Subtract(x=w874, y=4.5) -> (x-y=w873:dbl)
                n605 = Subtract(x=w885, y=40.5) -> (x-y=w876:dbl)
                n606 = vi-ref "goto.vi"() -> (w883:refnum<vi>)
                n607 = property class="VI"(reference=w883, error in=w877) -> ("Name"=w882:string)  [unwired: 2 out]
                n608 = Open VI Reference(type specifier VI Refnum (for type only)=refnum<vi> refnum, vi path=w882, options=128) -> (vi reference=w880:refnum<vi>)  [unwired: 3 in, 1 out]
                n609 = call-by-ref "Start Asynchronous Call"(reference=w880, "Y(mm)"=w873, "X(mm)"=w876) -> ()  [unwired: 10 in, 3 out]
              }
            }
          }
          event "B11": Value Change {
            n610 = event-data() -> ("NewVal"=w886:bool)  [unwired: 1 in, 5 out]
            n611 = property on="移动" class="Bool (strict)"() -> ("Value"=w889:bool)  [unwired: 2 in, 2 out]
            n612 = Not(x=w889) -> (.not. x?=w888:bool)
            n613 = And(x=w888, y=w886) -> (x .and. y?=w887:bool)
            n614 = case shown="True" w887 {
              frame False {
              }
              frame True {
                n615 = property on="A1-position-X" class="DigNum (strict)"() -> (error out=w895:errorcluster, "Value"=w902:dbl)  [unwired: 2 in, 1 out]
                n616 = property on="A1-position-Y" class="DigNum (strict)"(error in=w895) -> (error out=w894:errorcluster, "Value"=w891:dbl)  [unwired: 1 in, 1 out]
                n617 = Subtract(x=w891, y=4.5) -> (x-y=w890:dbl)
                n618 = Subtract(x=w902, y=45) -> (x-y=w893:dbl)
                n619 = vi-ref "goto.vi"() -> (w900:refnum<vi>)
                n620 = property class="VI"(reference=w900, error in=w894) -> ("Name"=w899:string)  [unwired: 2 out]
                n621 = Open VI Reference(type specifier VI Refnum (for type only)=refnum<vi> refnum, vi path=w899, options=128) -> (vi reference=w897:refnum<vi>)  [unwired: 3 in, 1 out]
                n622 = call-by-ref "Start Asynchronous Call"(reference=w897, "Y(mm)"=w890, "X(mm)"=w893) -> ()  [unwired: 10 in, 3 out]
              }
            }
          }
          event "B12": Value Change {
            n623 = event-data() -> ("NewVal"=w903:bool)  [unwired: 1 in, 5 out]
            n624 = property on="移动" class="Bool (strict)"() -> ("Value"=w906:bool)  [unwired: 2 in, 2 out]
            n625 = Not(x=w906) -> (.not. x?=w905:bool)
            n626 = And(x=w905, y=w903) -> (x .and. y?=w904:bool)
            n627 = case shown="True" w904 {
              frame False {
              }
              frame True {
                n628 = property on="A1-position-X" class="DigNum (strict)"() -> (error out=w912:errorcluster, "Value"=w919:dbl)  [unwired: 2 in, 1 out]
                n629 = property on="A1-position-Y" class="DigNum (strict)"(error in=w912) -> (error out=w911:errorcluster, "Value"=w908:dbl)  [unwired: 1 in, 1 out]
                n630 = Subtract(x=w908, y=4.5) -> (x-y=w907:dbl)
                n631 = Subtract(x=w919, y=49.5) -> (x-y=w910:dbl)
                n632 = vi-ref "goto.vi"() -> (w917:refnum<vi>)
                n633 = property class="VI"(reference=w917, error in=w911) -> ("Name"=w916:string)  [unwired: 2 out]
                n634 = Open VI Reference(type specifier VI Refnum (for type only)=refnum<vi> refnum, vi path=w916, options=128) -> (vi reference=w914:refnum<vi>)  [unwired: 3 in, 1 out]
                n635 = call-by-ref "Start Asynchronous Call"(reference=w914, "Y(mm)"=w907, "X(mm)"=w910) -> ()  [unwired: 10 in, 3 out]
              }
            }
          }
          event "C1": Value Change {
            n636 = event-data() -> ("NewVal"=w920:bool)  [unwired: 1 in, 5 out]
            n637 = property on="移动" class="Bool (strict)"() -> ("Value"=w923:bool)  [unwired: 2 in, 2 out]
            n638 = Not(x=w923) -> (.not. x?=w922:bool)
            n639 = And(x=w922, y=w920) -> (x .and. y?=w921:bool)
            n640 = case shown="True" w921 {
              frame False {
              }
              frame True {
                n641 = property on="A1-position-X" class="DigNum (strict)"() -> (error out=w929:errorcluster, "Value"=w936:dbl)  [unwired: 2 in, 1 out]
                n642 = property on="A1-position-Y" class="DigNum (strict)"(error in=w929) -> (error out=w928:errorcluster, "Value"=w925:dbl)  [unwired: 1 in, 1 out]
                n643 = Subtract(x=w925, y=9) -> (x-y=w924:dbl)
                n644 = Subtract(x=w936, y=0) -> (x-y=w927:dbl)
                n645 = vi-ref "goto.vi"() -> (w934:refnum<vi>)
                n646 = property class="VI"(reference=w934, error in=w928) -> ("Name"=w933:string)  [unwired: 2 out]
                n647 = Open VI Reference(type specifier VI Refnum (for type only)=refnum<vi> refnum, vi path=w933, options=128) -> (vi reference=w931:refnum<vi>)  [unwired: 3 in, 1 out]
                n648 = call-by-ref "Start Asynchronous Call"(reference=w931, "Y(mm)"=w924, "X(mm)"=w927) -> ()  [unwired: 10 in, 3 out]
              }
            }
          }
          event "C2": Value Change {
            n649 = event-data() -> ("NewVal"=w937:bool)  [unwired: 1 in, 5 out]
            n650 = property on="移动" class="Bool (strict)"() -> ("Value"=w940:bool)  [unwired: 2 in, 2 out]
            n651 = Not(x=w940) -> (.not. x?=w939:bool)
            n652 = And(x=w939, y=w937) -> (x .and. y?=w938:bool)
            n653 = case shown="True" w938 {
              frame False {
              }
              frame True {
                n654 = property on="A1-position-X" class="DigNum (strict)"() -> (error out=w946:errorcluster, "Value"=w953:dbl)  [unwired: 2 in, 1 out]
                n655 = property on="A1-position-Y" class="DigNum (strict)"(error in=w946) -> (error out=w945:errorcluster, "Value"=w942:dbl)  [unwired: 1 in, 1 out]
                n656 = Subtract(x=w942, y=9) -> (x-y=w941:dbl)
                n657 = Subtract(x=w953, y=4.5) -> (x-y=w944:dbl)
                n658 = vi-ref "goto.vi"() -> (w951:refnum<vi>)
                n659 = property class="VI"(reference=w951, error in=w945) -> ("Name"=w950:string)  [unwired: 2 out]
                n660 = Open VI Reference(type specifier VI Refnum (for type only)=refnum<vi> refnum, vi path=w950, options=128) -> (vi reference=w948:refnum<vi>)  [unwired: 3 in, 1 out]
                n661 = call-by-ref "Start Asynchronous Call"(reference=w948, "Y(mm)"=w941, "X(mm)"=w944) -> ()  [unwired: 10 in, 3 out]
              }
            }
          }
          event "C3": Value Change {
            n662 = event-data() -> ("NewVal"=w954:bool)  [unwired: 1 in, 5 out]
            n663 = property on="移动" class="Bool (strict)"() -> ("Value"=w957:bool)  [unwired: 2 in, 2 out]
            n664 = Not(x=w957) -> (.not. x?=w956:bool)
            n665 = And(x=w956, y=w954) -> (x .and. y?=w955:bool)
            n666 = case shown="True" w955 {
              frame False {
              }
              frame True {
                n667 = property on="A1-position-X" class="DigNum (strict)"() -> (error out=w963:errorcluster, "Value"=w970:dbl)  [unwired: 2 in, 1 out]
                n668 = property on="A1-position-Y" class="DigNum (strict)"(error in=w963) -> (error out=w962:errorcluster, "Value"=w959:dbl)  [unwired: 1 in, 1 out]
                n669 = Subtract(x=w959, y=9) -> (x-y=w958:dbl)
                n670 = Subtract(x=w970, y=9) -> (x-y=w961:dbl)
                n671 = vi-ref "goto.vi"() -> (w968:refnum<vi>)
                n672 = property class="VI"(reference=w968, error in=w962) -> ("Name"=w967:string)  [unwired: 2 out]
                n673 = Open VI Reference(type specifier VI Refnum (for type only)=refnum<vi> refnum, vi path=w967, options=128) -> (vi reference=w965:refnum<vi>)  [unwired: 3 in, 1 out]
                n674 = call-by-ref "Start Asynchronous Call"(reference=w965, "Y(mm)"=w958, "X(mm)"=w961) -> ()  [unwired: 10 in, 3 out]
              }
            }
          }
          event "C4": Value Change {
            n675 = event-data() -> ("NewVal"=w971:bool)  [unwired: 1 in, 5 out]
            n676 = property on="移动" class="Bool (strict)"() -> ("Value"=w974:bool)  [unwired: 2 in, 2 out]
            n677 = Not(x=w974) -> (.not. x?=w973:bool)
            n678 = And(x=w973, y=w971) -> (x .and. y?=w972:bool)
            n679 = case shown="True" w972 {
              frame False {
              }
              frame True {
                n680 = property on="A1-position-X" class="DigNum (strict)"() -> (error out=w980:errorcluster, "Value"=w987:dbl)  [unwired: 2 in, 1 out]
                n681 = property on="A1-position-Y" class="DigNum (strict)"(error in=w980) -> (error out=w979:errorcluster, "Value"=w976:dbl)  [unwired: 1 in, 1 out]
                n682 = Subtract(x=w976, y=9) -> (x-y=w975:dbl)
                n683 = Subtract(x=w987, y=13.5) -> (x-y=w978:dbl)
                n684 = vi-ref "goto.vi"() -> (w985:refnum<vi>)
                n685 = property class="VI"(reference=w985, error in=w979) -> ("Name"=w984:string)  [unwired: 2 out]
                n686 = Open VI Reference(type specifier VI Refnum (for type only)=refnum<vi> refnum, vi path=w984, options=128) -> (vi reference=w982:refnum<vi>)  [unwired: 3 in, 1 out]
                n687 = call-by-ref "Start Asynchronous Call"(reference=w982, "Y(mm)"=w975, "X(mm)"=w978) -> ()  [unwired: 10 in, 3 out]
              }
            }
          }
          event "C5": Value Change {
            n688 = event-data() -> ("NewVal"=w988:bool)  [unwired: 1 in, 5 out]
            n689 = property on="移动" class="Bool (strict)"() -> ("Value"=w991:bool)  [unwired: 2 in, 2 out]
            n690 = Not(x=w991) -> (.not. x?=w990:bool)
            n691 = And(x=w990, y=w988) -> (x .and. y?=w989:bool)
            n692 = case shown="True" w989 {
              frame False {
              }
              frame True {
                n693 = property on="A1-position-X" class="DigNum (strict)"() -> (error out=w997:errorcluster, "Value"=w1004:dbl)  [unwired: 2 in, 1 out]
                n694 = property on="A1-position-Y" class="DigNum (strict)"(error in=w997) -> (error out=w996:errorcluster, "Value"=w993:dbl)  [unwired: 1 in, 1 out]
                n695 = Subtract(x=w993, y=9) -> (x-y=w992:dbl)
                n696 = Subtract(x=w1004, y=18) -> (x-y=w995:dbl)
                n697 = vi-ref "goto.vi"() -> (w1002:refnum<vi>)
                n698 = property class="VI"(reference=w1002, error in=w996) -> ("Name"=w1001:string)  [unwired: 2 out]
                n699 = Open VI Reference(type specifier VI Refnum (for type only)=refnum<vi> refnum, vi path=w1001, options=128) -> (vi reference=w999:refnum<vi>)  [unwired: 3 in, 1 out]
                n700 = call-by-ref "Start Asynchronous Call"(reference=w999, "Y(mm)"=w992, "X(mm)"=w995) -> ()  [unwired: 10 in, 3 out]
              }
            }
          }
          event "C6": Value Change {
            n701 = event-data() -> ("NewVal"=w1005:bool)  [unwired: 1 in, 5 out]
            n702 = property on="移动" class="Bool (strict)"() -> ("Value"=w1008:bool)  [unwired: 2 in, 2 out]
            n703 = Not(x=w1008) -> (.not. x?=w1007:bool)
            n704 = And(x=w1007, y=w1005) -> (x .and. y?=w1006:bool)
            n705 = case shown="True" w1006 {
              frame False {
              }
              frame True {
                n706 = property on="A1-position-X" class="DigNum (strict)"() -> (error out=w1014:errorcluster, "Value"=w1021:dbl)  [unwired: 2 in, 1 out]
                n707 = property on="A1-position-Y" class="DigNum (strict)"(error in=w1014) -> (error out=w1013:errorcluster, "Value"=w1010:dbl)  [unwired: 1 in, 1 out]
                n708 = Subtract(x=w1010, y=9) -> (x-y=w1009:dbl)
                n709 = Subtract(x=w1021, y=22.5) -> (x-y=w1012:dbl)
                n710 = vi-ref "goto.vi"() -> (w1019:refnum<vi>)
                n711 = property class="VI"(reference=w1019, error in=w1013) -> ("Name"=w1018:string)  [unwired: 2 out]
                n712 = Open VI Reference(type specifier VI Refnum (for type only)=refnum<vi> refnum, vi path=w1018, options=128) -> (vi reference=w1016:refnum<vi>)  [unwired: 3 in, 1 out]
                n713 = call-by-ref "Start Asynchronous Call"(reference=w1016, "Y(mm)"=w1009, "X(mm)"=w1012) -> ()  [unwired: 10 in, 3 out]
              }
            }
          }
          event "C7": Value Change {
            n714 = event-data() -> ("NewVal"=w1022:bool)  [unwired: 1 in, 5 out]
            n715 = property on="移动" class="Bool (strict)"() -> ("Value"=w1025:bool)  [unwired: 2 in, 2 out]
            n716 = Not(x=w1025) -> (.not. x?=w1024:bool)
            n717 = And(x=w1024, y=w1022) -> (x .and. y?=w1023:bool)
            n718 = case shown="True" w1023 {
              frame False {
              }
              frame True {
                n719 = property on="A1-position-X" class="DigNum (strict)"() -> (error out=w1031:errorcluster, "Value"=w1038:dbl)  [unwired: 2 in, 1 out]
                n720 = property on="A1-position-Y" class="DigNum (strict)"(error in=w1031) -> (error out=w1030:errorcluster, "Value"=w1027:dbl)  [unwired: 1 in, 1 out]
                n721 = Subtract(x=w1027, y=9) -> (x-y=w1026:dbl)
                n722 = Subtract(x=w1038, y=27) -> (x-y=w1029:dbl)
                n723 = vi-ref "goto.vi"() -> (w1036:refnum<vi>)
                n724 = property class="VI"(reference=w1036, error in=w1030) -> ("Name"=w1035:string)  [unwired: 2 out]
                n725 = Open VI Reference(type specifier VI Refnum (for type only)=refnum<vi> refnum, vi path=w1035, options=128) -> (vi reference=w1033:refnum<vi>)  [unwired: 3 in, 1 out]
                n726 = call-by-ref "Start Asynchronous Call"(reference=w1033, "Y(mm)"=w1026, "X(mm)"=w1029) -> ()  [unwired: 10 in, 3 out]
              }
            }
          }
          event "C8": Value Change {
            n727 = event-data() -> ("NewVal"=w1039:bool)  [unwired: 1 in, 5 out]
            n728 = property on="移动" class="Bool (strict)"() -> ("Value"=w1042:bool)  [unwired: 2 in, 2 out]
            n729 = Not(x=w1042) -> (.not. x?=w1041:bool)
            n730 = And(x=w1041, y=w1039) -> (x .and. y?=w1040:bool)
            n731 = case shown="True" w1040 {
              frame False {
              }
              frame True {
                n732 = property on="A1-position-X" class="DigNum (strict)"() -> (error out=w1048:errorcluster, "Value"=w1055:dbl)  [unwired: 2 in, 1 out]
                n733 = property on="A1-position-Y" class="DigNum (strict)"(error in=w1048) -> (error out=w1047:errorcluster, "Value"=w1044:dbl)  [unwired: 1 in, 1 out]
                n734 = Subtract(x=w1044, y=9) -> (x-y=w1043:dbl)
                n735 = Subtract(x=w1055, y=31.5) -> (x-y=w1046:dbl)
                n736 = vi-ref "goto.vi"() -> (w1053:refnum<vi>)
                n737 = property class="VI"(reference=w1053, error in=w1047) -> ("Name"=w1052:string)  [unwired: 2 out]
                n738 = Open VI Reference(type specifier VI Refnum (for type only)=refnum<vi> refnum, vi path=w1052, options=128) -> (vi reference=w1050:refnum<vi>)  [unwired: 3 in, 1 out]
                n739 = call-by-ref "Start Asynchronous Call"(reference=w1050, "Y(mm)"=w1043, "X(mm)"=w1046) -> ()  [unwired: 10 in, 3 out]
              }
            }
          }
          event "C9": Value Change {
            n740 = event-data() -> ("NewVal"=w1056:bool)  [unwired: 1 in, 5 out]
            n741 = property on="移动" class="Bool (strict)"() -> ("Value"=w1059:bool)  [unwired: 2 in, 2 out]
            n742 = Not(x=w1059) -> (.not. x?=w1058:bool)
            n743 = And(x=w1058, y=w1056) -> (x .and. y?=w1057:bool)
            n744 = case shown="True" w1057 {
              frame False {
              }
              frame True {
                n745 = property on="A1-position-X" class="DigNum (strict)"() -> (error out=w1065:errorcluster, "Value"=w1072:dbl)  [unwired: 2 in, 1 out]
                n746 = property on="A1-position-Y" class="DigNum (strict)"(error in=w1065) -> (error out=w1064:errorcluster, "Value"=w1061:dbl)  [unwired: 1 in, 1 out]
                n747 = Subtract(x=w1061, y=9) -> (x-y=w1060:dbl)
                n748 = Subtract(x=w1072, y=36) -> (x-y=w1063:dbl)
                n749 = vi-ref "goto.vi"() -> (w1070:refnum<vi>)
                n750 = property class="VI"(reference=w1070, error in=w1064) -> ("Name"=w1069:string)  [unwired: 2 out]
                n751 = Open VI Reference(type specifier VI Refnum (for type only)=refnum<vi> refnum, vi path=w1069, options=128) -> (vi reference=w1067:refnum<vi>)  [unwired: 3 in, 1 out]
                n752 = call-by-ref "Start Asynchronous Call"(reference=w1067, "Y(mm)"=w1060, "X(mm)"=w1063) -> ()  [unwired: 10 in, 3 out]
              }
            }
          }
          event "C10": Value Change {
            n753 = event-data() -> ("NewVal"=w1073:bool)  [unwired: 1 in, 5 out]
            n754 = property on="移动" class="Bool (strict)"() -> ("Value"=w1076:bool)  [unwired: 2 in, 2 out]
            n755 = Not(x=w1076) -> (.not. x?=w1075:bool)
            n756 = And(x=w1075, y=w1073) -> (x .and. y?=w1074:bool)
            n757 = case shown="True" w1074 {
              frame False {
              }
              frame True {
                n758 = property on="A1-position-X" class="DigNum (strict)"() -> (error out=w1082:errorcluster, "Value"=w1089:dbl)  [unwired: 2 in, 1 out]
                n759 = property on="A1-position-Y" class="DigNum (strict)"(error in=w1082) -> (error out=w1081:errorcluster, "Value"=w1078:dbl)  [unwired: 1 in, 1 out]
                n760 = Subtract(x=w1078, y=9) -> (x-y=w1077:dbl)
                n761 = Subtract(x=w1089, y=40.5) -> (x-y=w1080:dbl)
                n762 = vi-ref "goto.vi"() -> (w1087:refnum<vi>)
                n763 = property class="VI"(reference=w1087, error in=w1081) -> ("Name"=w1086:string)  [unwired: 2 out]
                n764 = Open VI Reference(type specifier VI Refnum (for type only)=refnum<vi> refnum, vi path=w1086, options=128) -> (vi reference=w1084:refnum<vi>)  [unwired: 3 in, 1 out]
                n765 = call-by-ref "Start Asynchronous Call"(reference=w1084, "Y(mm)"=w1077, "X(mm)"=w1080) -> ()  [unwired: 10 in, 3 out]
              }
            }
          }
          event "C11": Value Change {
            n766 = event-data() -> ("NewVal"=w1090:bool)  [unwired: 1 in, 5 out]
            n767 = property on="移动" class="Bool (strict)"() -> ("Value"=w1093:bool)  [unwired: 2 in, 2 out]
            n768 = Not(x=w1093) -> (.not. x?=w1092:bool)
            n769 = And(x=w1092, y=w1090) -> (x .and. y?=w1091:bool)
            n770 = case shown="True" w1091 {
              frame False {
              }
              frame True {
                n771 = property on="A1-position-X" class="DigNum (strict)"() -> (error out=w1099:errorcluster, "Value"=w1106:dbl)  [unwired: 2 in, 1 out]
                n772 = property on="A1-position-Y" class="DigNum (strict)"(error in=w1099) -> (error out=w1098:errorcluster, "Value"=w1095:dbl)  [unwired: 1 in, 1 out]
                n773 = Subtract(x=w1095, y=9) -> (x-y=w1094:dbl)
                n774 = Subtract(x=w1106, y=45) -> (x-y=w1097:dbl)
                n775 = vi-ref "goto.vi"() -> (w1104:refnum<vi>)
                n776 = property class="VI"(reference=w1104, error in=w1098) -> ("Name"=w1103:string)  [unwired: 2 out]
                n777 = Open VI Reference(type specifier VI Refnum (for type only)=refnum<vi> refnum, vi path=w1103, options=128) -> (vi reference=w1101:refnum<vi>)  [unwired: 3 in, 1 out]
                n778 = call-by-ref "Start Asynchronous Call"(reference=w1101, "Y(mm)"=w1094, "X(mm)"=w1097) -> ()  [unwired: 10 in, 3 out]
              }
            }
          }
          event "C12": Value Change {
            n779 = event-data() -> ("NewVal"=w1107:bool)  [unwired: 1 in, 5 out]
            n780 = property on="移动" class="Bool (strict)"() -> ("Value"=w1110:bool)  [unwired: 2 in, 2 out]
            n781 = Not(x=w1110) -> (.not. x?=w1109:bool)
            n782 = And(x=w1109, y=w1107) -> (x .and. y?=w1108:bool)
            n783 = case shown="True" w1108 {
              frame False {
              }
              frame True {
                n784 = property on="A1-position-X" class="DigNum (strict)"() -> (error out=w1116:errorcluster, "Value"=w1123:dbl)  [unwired: 2 in, 1 out]
                n785 = property on="A1-position-Y" class="DigNum (strict)"(error in=w1116) -> (error out=w1115:errorcluster, "Value"=w1112:dbl)  [unwired: 1 in, 1 out]
                n786 = Subtract(x=w1112, y=9) -> (x-y=w1111:dbl)
                n787 = Subtract(x=w1123, y=49.5) -> (x-y=w1114:dbl)
                n788 = vi-ref "goto.vi"() -> (w1121:refnum<vi>)
                n789 = property class="VI"(reference=w1121, error in=w1115) -> ("Name"=w1120:string)  [unwired: 2 out]
                n790 = Open VI Reference(type specifier VI Refnum (for type only)=refnum<vi> refnum, vi path=w1120, options=128) -> (vi reference=w1118:refnum<vi>)  [unwired: 3 in, 1 out]
                n791 = call-by-ref "Start Asynchronous Call"(reference=w1118, "Y(mm)"=w1111, "X(mm)"=w1114) -> ()  [unwired: 10 in, 3 out]
              }
            }
          }
          event "D1": Value Change {
            n792 = event-data() -> ("NewVal"=w1124:bool)  [unwired: 1 in, 5 out]
            n793 = property on="移动" class="Bool (strict)"() -> ("Value"=w1127:bool)  [unwired: 2 in, 2 out]
            n794 = Not(x=w1127) -> (.not. x?=w1126:bool)
            n795 = And(x=w1126, y=w1124) -> (x .and. y?=w1125:bool)
            n796 = case shown="True" w1125 {
              frame False {
              }
              frame True {
                n797 = property on="A1-position-X" class="DigNum (strict)"() -> (error out=w1133:errorcluster, "Value"=w1140:dbl)  [unwired: 2 in, 1 out]
                n798 = property on="A1-position-Y" class="DigNum (strict)"(error in=w1133) -> (error out=w1132:errorcluster, "Value"=w1129:dbl)  [unwired: 1 in, 1 out]
                n799 = Subtract(x=w1129, y=13.5) -> (x-y=w1128:dbl)
                n800 = Subtract(x=w1140, y=0) -> (x-y=w1131:dbl)
                n801 = vi-ref "goto.vi"() -> (w1138:refnum<vi>)
                n802 = property class="VI"(reference=w1138, error in=w1132) -> ("Name"=w1137:string)  [unwired: 2 out]
                n803 = Open VI Reference(type specifier VI Refnum (for type only)=refnum<vi> refnum, vi path=w1137, options=128) -> (vi reference=w1135:refnum<vi>)  [unwired: 3 in, 1 out]
                n804 = call-by-ref "Start Asynchronous Call"(reference=w1135, "Y(mm)"=w1128, "X(mm)"=w1131) -> ()  [unwired: 10 in, 3 out]
              }
            }
          }
          event "D2": Value Change {
            n805 = event-data() -> ("NewVal"=w1141:bool)  [unwired: 1 in, 5 out]
            n806 = property on="移动" class="Bool (strict)"() -> ("Value"=w1144:bool)  [unwired: 2 in, 2 out]
            n807 = Not(x=w1144) -> (.not. x?=w1143:bool)
            n808 = And(x=w1143, y=w1141) -> (x .and. y?=w1142:bool)
            n809 = case shown="True" w1142 {
              frame False {
              }
              frame True {
                n810 = property on="A1-position-X" class="DigNum (strict)"() -> (error out=w1150:errorcluster, "Value"=w1157:dbl)  [unwired: 2 in, 1 out]
                n811 = property on="A1-position-Y" class="DigNum (strict)"(error in=w1150) -> (error out=w1149:errorcluster, "Value"=w1146:dbl)  [unwired: 1 in, 1 out]
                n812 = Subtract(x=w1146, y=13.5) -> (x-y=w1145:dbl)
                n813 = Subtract(x=w1157, y=4.5) -> (x-y=w1148:dbl)
                n814 = vi-ref "goto.vi"() -> (w1155:refnum<vi>)
                n815 = property class="VI"(reference=w1155, error in=w1149) -> ("Name"=w1154:string)  [unwired: 2 out]
                n816 = Open VI Reference(type specifier VI Refnum (for type only)=refnum<vi> refnum, vi path=w1154, options=128) -> (vi reference=w1152:refnum<vi>)  [unwired: 3 in, 1 out]
                n817 = call-by-ref "Start Asynchronous Call"(reference=w1152, "Y(mm)"=w1145, "X(mm)"=w1148) -> ()  [unwired: 10 in, 3 out]
              }
            }
          }
          event "D3": Value Change {
            n818 = event-data() -> ("NewVal"=w1158:bool)  [unwired: 1 in, 5 out]
            n819 = property on="移动" class="Bool (strict)"() -> ("Value"=w1161:bool)  [unwired: 2 in, 2 out]
            n820 = Not(x=w1161) -> (.not. x?=w1160:bool)
            n821 = And(x=w1160, y=w1158) -> (x .and. y?=w1159:bool)
            n822 = case shown="True" w1159 {
              frame False {
              }
              frame True {
                n823 = property on="A1-position-X" class="DigNum (strict)"() -> (error out=w1167:errorcluster, "Value"=w1174:dbl)  [unwired: 2 in, 1 out]
                n824 = property on="A1-position-Y" class="DigNum (strict)"(error in=w1167) -> (error out=w1166:errorcluster, "Value"=w1163:dbl)  [unwired: 1 in, 1 out]
                n825 = Subtract(x=w1163, y=13.5) -> (x-y=w1162:dbl)
                n826 = Subtract(x=w1174, y=9) -> (x-y=w1165:dbl)
                n827 = vi-ref "goto.vi"() -> (w1172:refnum<vi>)
                n828 = property class="VI"(reference=w1172, error in=w1166) -> ("Name"=w1171:string)  [unwired: 2 out]
                n829 = Open VI Reference(type specifier VI Refnum (for type only)=refnum<vi> refnum, vi path=w1171, options=128) -> (vi reference=w1169:refnum<vi>)  [unwired: 3 in, 1 out]
                n830 = call-by-ref "Start Asynchronous Call"(reference=w1169, "Y(mm)"=w1162, "X(mm)"=w1165) -> ()  [unwired: 10 in, 3 out]
              }
            }
          }
          event "D4": Value Change {
            n831 = event-data() -> ("NewVal"=w1175:bool)  [unwired: 1 in, 5 out]
            n832 = property on="移动" class="Bool (strict)"() -> ("Value"=w1178:bool)  [unwired: 2 in, 2 out]
            n833 = Not(x=w1178) -> (.not. x?=w1177:bool)
            n834 = And(x=w1177, y=w1175) -> (x .and. y?=w1176:bool)
            n835 = case shown="True" w1176 {
              frame False {
              }
              frame True {
                n836 = property on="A1-position-X" class="DigNum (strict)"() -> (error out=w1184:errorcluster, "Value"=w1191:dbl)  [unwired: 2 in, 1 out]
                n837 = property on="A1-position-Y" class="DigNum (strict)"(error in=w1184) -> (error out=w1183:errorcluster, "Value"=w1180:dbl)  [unwired: 1 in, 1 out]
                n838 = Subtract(x=w1180, y=13.5) -> (x-y=w1179:dbl)
                n839 = Subtract(x=w1191, y=13.5) -> (x-y=w1182:dbl)
                n840 = vi-ref "goto.vi"() -> (w1189:refnum<vi>)
                n841 = property class="VI"(reference=w1189, error in=w1183) -> ("Name"=w1188:string)  [unwired: 2 out]
                n842 = Open VI Reference(type specifier VI Refnum (for type only)=refnum<vi> refnum, vi path=w1188, options=128) -> (vi reference=w1186:refnum<vi>)  [unwired: 3 in, 1 out]
                n843 = call-by-ref "Start Asynchronous Call"(reference=w1186, "Y(mm)"=w1179, "X(mm)"=w1182) -> ()  [unwired: 10 in, 3 out]
              }
            }
          }
          event "D5": Value Change {
            n844 = event-data() -> ("NewVal"=w1192:bool)  [unwired: 1 in, 5 out]
            n845 = property on="移动" class="Bool (strict)"() -> ("Value"=w1195:bool)  [unwired: 2 in, 2 out]
            n846 = Not(x=w1195) -> (.not. x?=w1194:bool)
            n847 = And(x=w1194, y=w1192) -> (x .and. y?=w1193:bool)
            n848 = case shown="True" w1193 {
              frame False {
              }
              frame True {
                n849 = property on="A1-position-X" class="DigNum (strict)"() -> (error out=w1201:errorcluster, "Value"=w1208:dbl)  [unwired: 2 in, 1 out]
                n850 = property on="A1-position-Y" class="DigNum (strict)"(error in=w1201) -> (error out=w1200:errorcluster, "Value"=w1197:dbl)  [unwired: 1 in, 1 out]
                n851 = Subtract(x=w1197, y=13.5) -> (x-y=w1196:dbl)
                n852 = Subtract(x=w1208, y=18) -> (x-y=w1199:dbl)
                n853 = vi-ref "goto.vi"() -> (w1206:refnum<vi>)
                n854 = property class="VI"(reference=w1206, error in=w1200) -> ("Name"=w1205:string)  [unwired: 2 out]
                n855 = Open VI Reference(type specifier VI Refnum (for type only)=refnum<vi> refnum, vi path=w1205, options=128) -> (vi reference=w1203:refnum<vi>)  [unwired: 3 in, 1 out]
                n856 = call-by-ref "Start Asynchronous Call"(reference=w1203, "Y(mm)"=w1196, "X(mm)"=w1199) -> ()  [unwired: 10 in, 3 out]
              }
            }
          }
          event "D6": Value Change {
            n857 = event-data() -> ("NewVal"=w1209:bool)  [unwired: 1 in, 5 out]
            n858 = property on="移动" class="Bool (strict)"() -> ("Value"=w1212:bool)  [unwired: 2 in, 2 out]
            n859 = Not(x=w1212) -> (.not. x?=w1211:bool)
            n860 = And(x=w1211, y=w1209) -> (x .and. y?=w1210:bool)
            n861 = case shown="True" w1210 {
              frame False {
              }
              frame True {
                n862 = property on="A1-position-X" class="DigNum (strict)"() -> (error out=w1218:errorcluster, "Value"=w1225:dbl)  [unwired: 2 in, 1 out]
                n863 = property on="A1-position-Y" class="DigNum (strict)"(error in=w1218) -> (error out=w1217:errorcluster, "Value"=w1214:dbl)  [unwired: 1 in, 1 out]
                n864 = Subtract(x=w1214, y=13.5) -> (x-y=w1213:dbl)
                n865 = Subtract(x=w1225, y=22.5) -> (x-y=w1216:dbl)
                n866 = vi-ref "goto.vi"() -> (w1223:refnum<vi>)
                n867 = property class="VI"(reference=w1223, error in=w1217) -> ("Name"=w1222:string)  [unwired: 2 out]
                n868 = Open VI Reference(type specifier VI Refnum (for type only)=refnum<vi> refnum, vi path=w1222, options=128) -> (vi reference=w1220:refnum<vi>)  [unwired: 3 in, 1 out]
                n869 = call-by-ref "Start Asynchronous Call"(reference=w1220, "Y(mm)"=w1213, "X(mm)"=w1216) -> ()  [unwired: 10 in, 3 out]
              }
            }
          }
          event "D7": Value Change {
            n870 = event-data() -> ("NewVal"=w1226:bool)  [unwired: 1 in, 5 out]
            n871 = property on="移动" class="Bool (strict)"() -> ("Value"=w1229:bool)  [unwired: 2 in, 2 out]
            n872 = Not(x=w1229) -> (.not. x?=w1228:bool)
            n873 = And(x=w1228, y=w1226) -> (x .and. y?=w1227:bool)
            n874 = case shown="True" w1227 {
              frame False {
              }
              frame True {
                n875 = property on="A1-position-X" class="DigNum (strict)"() -> (error out=w1235:errorcluster, "Value"=w1242:dbl)  [unwired: 2 in, 1 out]
                n876 = property on="A1-position-Y" class="DigNum (strict)"(error in=w1235) -> (error out=w1234:errorcluster, "Value"=w1231:dbl)  [unwired: 1 in, 1 out]
                n877 = Subtract(x=w1231, y=13.5) -> (x-y=w1230:dbl)
                n878 = Subtract(x=w1242, y=27) -> (x-y=w1233:dbl)
                n879 = vi-ref "goto.vi"() -> (w1240:refnum<vi>)
                n880 = property class="VI"(reference=w1240, error in=w1234) -> ("Name"=w1239:string)  [unwired: 2 out]
                n881 = Open VI Reference(type specifier VI Refnum (for type only)=refnum<vi> refnum, vi path=w1239, options=128) -> (vi reference=w1237:refnum<vi>)  [unwired: 3 in, 1 out]
                n882 = call-by-ref "Start Asynchronous Call"(reference=w1237, "Y(mm)"=w1230, "X(mm)"=w1233) -> ()  [unwired: 10 in, 3 out]
              }
            }
          }
          event "ShutDownSystem": Value Change {
            n883 = event-data() -> ("NewVal"=w1244:bool)  [unwired: 1 in, 5 out]
            n884 = case shown="True" w1244 {
              tunnel: w1243 -> [_ w1248]
              frame False {
              }
              frame True {
                n885 = Unbundle By Name(w1248) -> ("ConfiguredPumpCom"=w1247:refnum<visa-resource-name>, "ConfiguredLaserCom"=w1246:refnum<visa-resource-name>)
                n886 = VISA Close(VISA resource name=w1247) -> (error out=w1245:errorcluster)  [unwired: 1 in]
                n887 = VISA Close(VISA resource name=w1246, error in (no error)=w1245) -> ()  [unwired: 1 out]
              }
            }
          }
        }
      }
    }
  }
  n888 = flat-sequence {
    tunnel: w18 -> [w1252]
    frame #0 {
      n889 = Unbundle(w1252) -> ("tasks"=w1251:T10, "interface"=w1250:T9, "error out"=w1249:errorcluster)
      n890 = call "USB6343_Control_v1.6.2.vi"("error in"=w1249, "interface"=w1250, "tasks"=w1251) -> ()  [unwired: 9 in]
    }
    frame #1 {
      n891 = call "setDO.vi"("channel"=15, "on/off"=TRUE) -> ("错误输出"=w1256:errorcluster)  [unwired: 9 in]
      n892 = flat-sequence {
        tunnel: w1256 -> [w1259]
        tunnel: [w1259] -> _
        tunnel: [w1259] -> w1253
        frame #0 {
          n893 = Wait (ms)(milliseconds to wait=u32 1000) -> ()  [unwired: 1 out]
        }
      }
      n894 = call "setDO.vi"("错误输入（无错误）"=w1253, "channel"=15, "on/off"=FALSE) -> ()  [unwired: 8 in, 1 out]
    }
  }
  n895 = while {
    tunnel: w20 -> [w1288]
    tunnel: w19 -> [w1286]
    stop <- FALSE stop-if-true
    n896 = Unbundle By Name(w1288) -> ("pump semaphore"=w1287:T2, "laser semaphore"=w1283:T2)
    n897 = Unbundle By Name(w1286) -> ("ConfiguredPumpCom"=w1285:refnum<visa-resource-name>, "ConfiguredLaserCom"=w1269:refnum<visa-resource-name>)
    n898 = call <vilib>:"Acquire Semaphore.vi"("semaphore"=w1287) -> ("error out"=w1268:errorcluster, "semaphore out"=w1284:T2)  [unwired: 4 in, 1 out]
    n899 = call "pumpStatus.vi"("VISA resource name"=w1285, "error in (no error)"=w1268) -> ("PumpKW"=→"PumpKW":dbl, "PumpTemp"=→"PumpTemp":u16, "PumpAmps"=→"PumpAmps":dbl, "PumpVolts"=→"PumpVolts":dbl, "TurboSpeed"=→"TurboSpeed":dbl, "error out"=w1267:errorcluster)  [unwired: 8 in]
    n900 = call <vilib>:"Release Semaphore.vi"("error in (no error)"=w1267, "semaphore"=w1284) -> ("error out"=w1261:errorcluster)  [unwired: 4 in, 1 out]
    n901 = call <vilib>:"Acquire Semaphore.vi"("error in (no error)"=w1261, "semaphore"=w1283) -> ("error out"=w1266:errorcluster, "semaphore out"=w1282:T2)  [unwired: 3 in, 1 out]
    n902 = call "Laser-Get-Shotstatus.vi"("VISA resource name"=w1269, "error in (no error)"=w1266) -> ("VISA resource name out"=w1265:refnum<visa-resource-name>, "cluster"=→"cluster":T6, "error out"=w1263:errorcluster)
    n903 = flat-sequence {
      tunnel: [w1289] -> w1262
      tunnel: w1263 -> [w1289]
      frame #0 {
        n904 = Wait (ms)(milliseconds to wait=50) -> ()  [unwired: 1 out]
      }
    }
    n905 = call "Laser-Set-Parmeter.vi"("error in (no error)"=w1262, "LaserHV"="LaserHV", "LaserFreq"="频率/Hz", "SetLaserEnergy"="SetLaserEnergy", "VISA resource name"=w1265) -> ("error out"=w1264:errorcluster)  [unwired: 1 in, 1 out]
    n906 = call <vilib>:"Release Semaphore.vi"("error in (no error)"=w1264, "semaphore"=w1282) -> ("error out"=w1281:errorcluster)  [unwired: 4 in, 1 out]
    n907 = call "Time Delay2"("error in (no error)"=w1281, "Delay Time (s)"=0.3) -> ()  [unwired: 9 in, 1 out]
  }
  n908 = call <vilib>:"IMAQdx Enumerate Cameras.vi"() -> ("error out"=w9:errorcluster, "Camera Information Array"=w6:T14)  [unwired: 10 in]
  n909 = Index Array(array=w6, index=0) -> (element=w8:T15)
  n910 = Unbundle By Name(w8) -> ("InterfaceName"=w16:string)
  n911 = call <vilib>:"IMAQdx Open Camera.vi"("error in"=w9, "Session In"=w16) -> ("error out"=w3:errorcluster, "Session Out"=w4:T16)  [unwired: 8 in]
  n912 = property class="IMAQdx" props=["VideoMode", "Width", "Height"](reference=w4, error in=w3, "VideoMode"=u32 13) -> (reference out=w2:T16, error out=w1:errorcluster)  [unwired: 2 out]
  n913 = call "IMAQ Create"("Image Name"=w16) -> ("New Image"=w11:T1)  [unwired: 4 in, 1 out]
  n914 = call <vilib>:"IMAQdx Configure Grab.vi"("error in"=w1, "Session In"=w2) -> ("error out"=w15:errorcluster, "Session Out"=w10:T16)  [unwired: 8 in]
  n915 = while {
    tunnel: w15 -> [w1297]
    tunnel: w10 -> [w1296]
    tunnel: w11 -> [w1295]
    tunnel: [w1294] -> w12
    tunnel: [w1293] -> w13
    tunnel: [w1292] -> w14
    stop <- FALSE stop-if-true
    n916 = call <vilib>:"IMAQdx Grab.vi"("error in"=w1297, "Image In"=w1295, "Session In"=w1296) -> ("error out"=w1294:errorcluster, "Image Out"=w1292:T1, "Session Out"=w1293:T16)  [unwired: 5 in, 1 out]
    "Image" <- w1292
  }
  n917 = call "IMAQ Dispose"("Image"=w14) -> ()  [unwired: 5 in, 1 out]
  n918 = call <vilib>:"IMAQdx Close Camera.vi"("error in"=w12, "Session In"=w13) -> ()  [unwired: 9 in, 1 out]
